vi "attenuation meter.vi"() -> ()   [LabVIEW 2014]
uses:
  Controls/App Data.ctl
  Controls/Main Enum.ctl
  <vilib>/Utility/NIReport.llb/NI_ReportGenerationCore.lvlib
  <resource>/objmgr/daqmx.rc
panel:
  in  "Erase all plots":bool
  out "Test results (spec.)":string
  in  "show test details":bool
  out "detailed results":string
  in  "Select TWT specification":string(combo)
  in  "auto measurement":bool
  in  "Number of cursors per plot":i32=4 min=2 max=4
  in  "plot 2 cursors visible?":bool=TRUE
  in  "plot 3 cursors visible?":bool=TRUE
  in  "plot 1 cursors visible?":bool=TRUE
  in  "Select plot":T1(radio)
  in  "Plot 3 color":u32(colorbox)=393471 caption="Plot 3"
  in  "Plot 2 color":u32(colorbox)=16716306 caption="Plot 2"
  in  "Plot 1 color":u32(colorbox) caption="Plot 1"
  in  "RF meter max.":dbl=10.1 min=0.0 max=500.0 format="%.2g"
  in  "RF meter min.":dbl=7.5 min=0.0 max=500.0 format="%.2g"
  in  "Batch":string="Batch: "
  in  "Run No":string="Run No: "
  in  "Date":string
  in  "Tube Type":string="Tube Type: "
  in  "Auto Record":bool
  in  "Device status":bool
  out "0 dB att. voltage (during last calibration)":dbl format="%.3g"
  out "Input voltages (updates \nonly when recording)":T2 {"Stop switch voltage" format="%.3g"; "Start switch voltage" format="%.3g"; "position voltage" format="%.3g"; "RF out voltage" format="%.3g"}
  in  "Re-calibrate 0dB":bool
  in  "Erase plot":bool
  in  "Record":bool
  in  "Print Button":bool
  in  "Select printer":string(combo)
  in  "minimum y [dB]":dbl=-1.0 min=-100.0 max=-0.1 step=0.1 format="%.1g"
  in  "averaging (1-10)":i32=5 min=1 max=10 step=1
  in  "ref. line [dB]":dbl=-0.09999999999999991 min=-5.0 max=0.0 step=0.01 format="%.3f"
  out "error out 2":errorcluster
  in  "error out":errorcluster
  out "XY Graph":T3(graph)
  # "Settings"
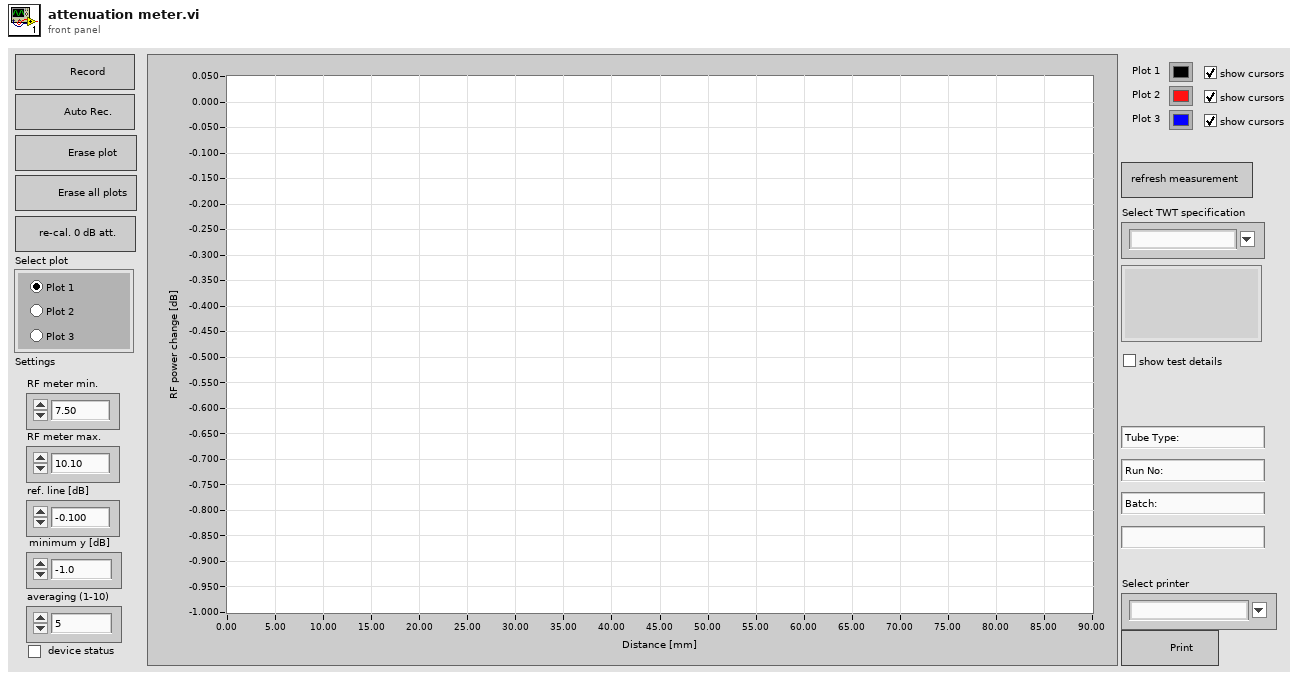
[diagram p1: front panel]
types:
  T1 = enum32{"Radio Selection 1", "Radio Selection 2", "Radio Selection 3"}
  T2 = cluster{"RF out voltage":dbl, "position voltage":dbl, "Start switch voltage":dbl, "Stop switch voltage":dbl}
  T3 = cluster{"plot 1 data":dbl[], "plot 1 data":dbl[]}[]
  T4 = typedef "Main Enum.ctl" = enum16{"Idle", "Initialize 1", "Initialize 2", "Initialize 3", "Calibrate RF output", "Update peaks colours", "Update anott. plots", "Save results", "Load results", "Erase plot", "Erase all plots", "Read new data", "Update plots", "Peak attenuation meas.", "Auto measurement", "Update cursors", "Update all cursors", "Print", "Check Start Stop triggers", "Plot 1 cursors visibility", "Plot 2 cursors visibility", "Plot 3 cursors visibility", "Error handler", "Exit", "Check results (spec.)"}
  T5 = typedef "App Data.ctl" = cluster{"DAQmx Task Name":refnum<k21>, "plot 0 data (ref.)":dbl[][], "plot 1 data":dbl[][], "plot 2 data":dbl[][], "plot 3 data":dbl[][], "Anott. plots":cluster{"plot 4 (anott.)":cluster{"x":dbl[], "y":dbl[]}, "plot 5 (anott.)":cluster{"x":dbl[], "y":dbl[]}, "plot 6 (anott.)":cluster{"x":dbl[], "y":dbl[]}}, "Active plot":u32, "Recording?":bool, "Cursors per plot":i32}
  T6 = enum16{"read", "write", "write number of cursors per plot only"}
  T7 = enum16{"get TWT types", "read TWT spec.", "save TWT spec."}
  T8 = enum8{"Enabled", "Disabled", "Disabled and Grayed Out"}
  T9 = enum16{"get TWT types", "read TWT spec.", "save TWT spec.", "remove TWT spec."}
  T10 = cluster{"plot 1 cursors visible? ":bool, "plot 2 cursors visible?":bool, "plot 3 cursors visible?":bool, "No of cursors per plot":i32}
  T11 = enum32{"invalid app kind", "Development System", "Run Time System", "Student Edition", "Embedded LabVIEW", "Evaluation", "Custom"}
  T12 = cluster{"plot 4 (anott.)":cluster{"x":dbl[], "y":dbl[]}, "plot 5 (anott.)":cluster{"x":dbl[], "y":dbl[]}, "plot 6 (anott.)":cluster{"x":dbl[], "y":dbl[]}}
  T13 = typedef "TWT spec..ctl" = cluster{"Reference level":dbl, "L1 min":dbl, "L1 max":dbl, "L2 min":dbl, "L2 max":dbl, "L3 min":dbl, "L3 max":dbl, "Tip loss nominal":dbl, "Tip loss min":dbl, "Tip loss max":dbl, "Centre loss nominal":dbl, "Centre loss min":dbl, "Centre loss max":dbl}
  T14 = cluster{"plot 3 data":dbl[], "plot 3 data":dbl[]}[]
  T15 = typedef "dist. between cursors.ctl" = cluster{"0 to c1":dbl, "c1 to c2":dbl, "c1 to c3":dbl, "c3 to c4":dbl}
  T16 = cluster{"Plot 1 distances":T15, "Plot 2 distances":T15, "Plot 3 distances":T15}
  T17 = cluster{"Tube Type":string, "Date":string, "Run No":string, "Batch":string}
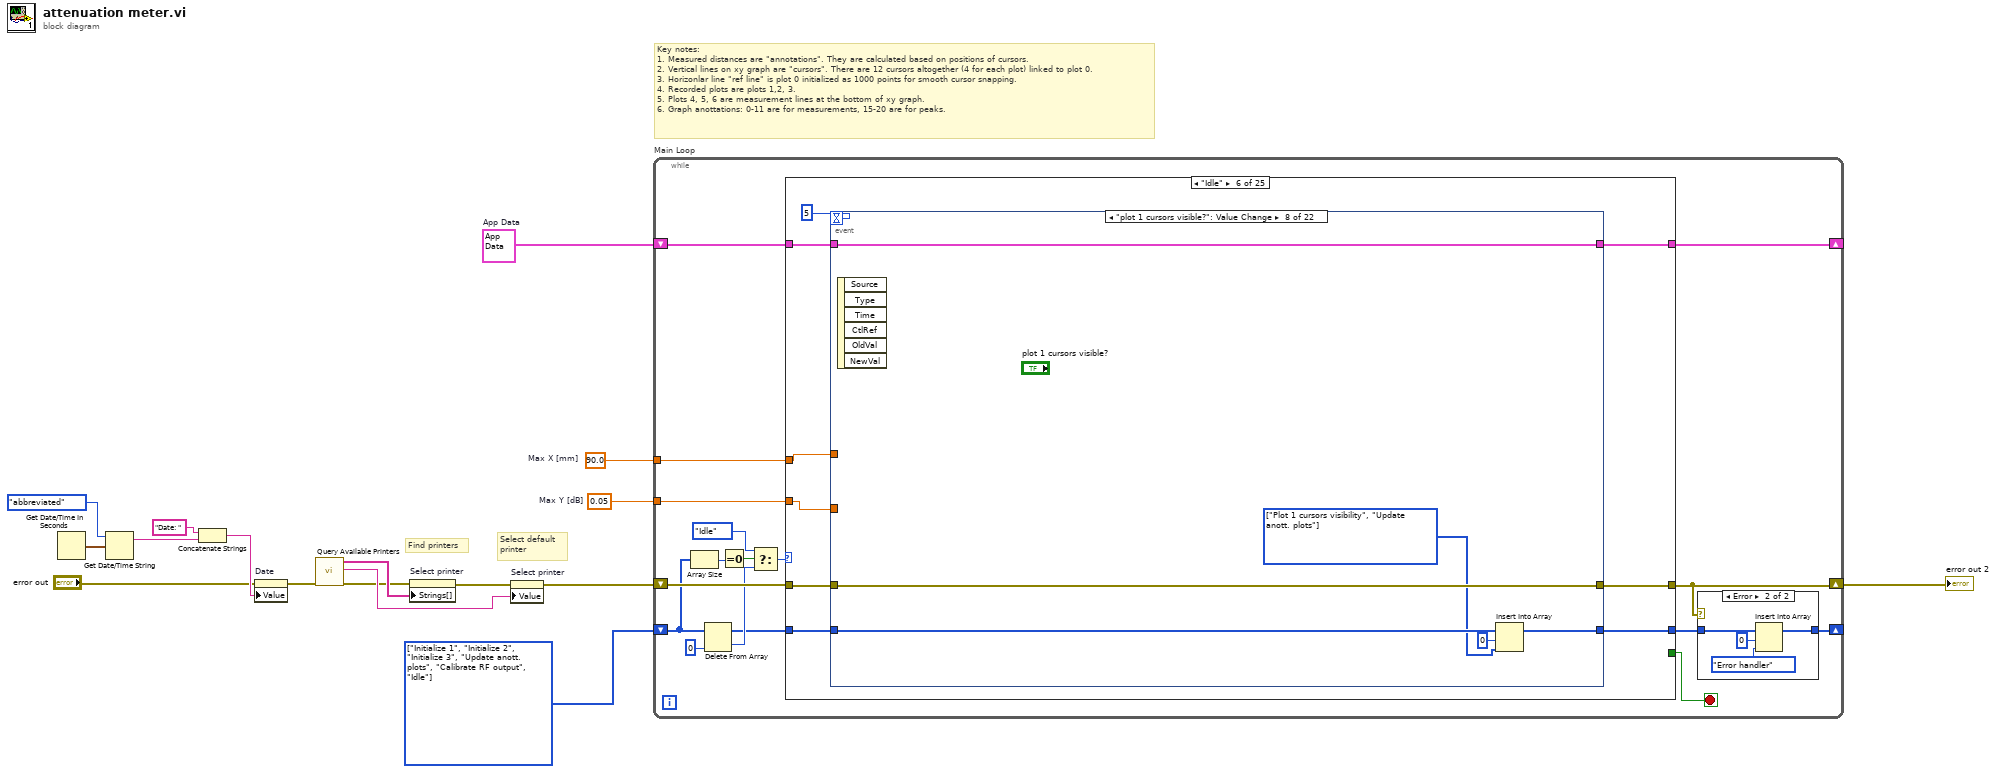
[diagram p0: block diagram]
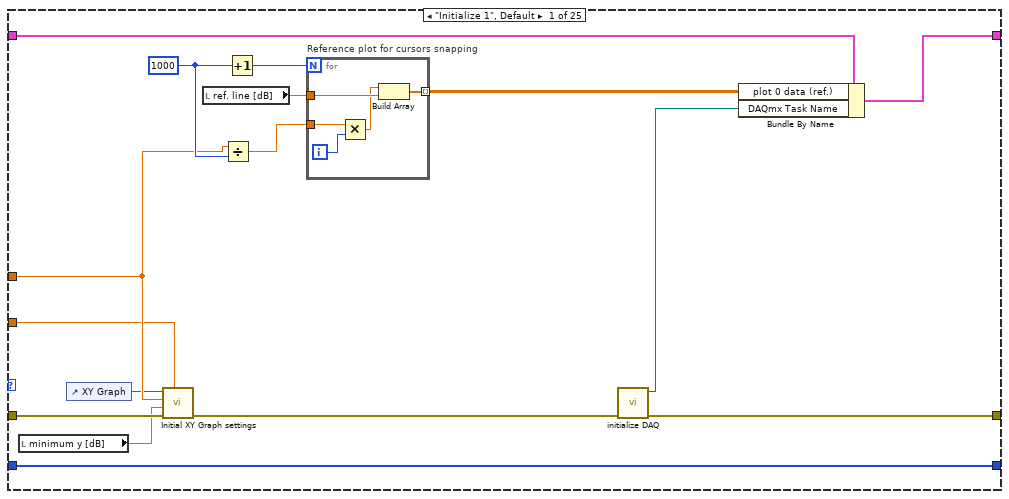
[diagram p3: hidden frame]
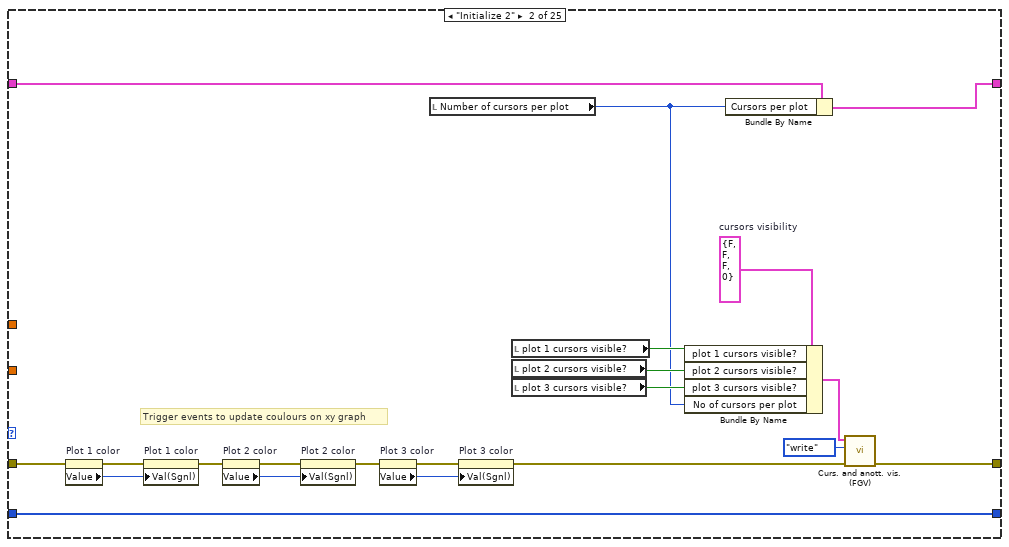
[diagram p4: hidden frame]
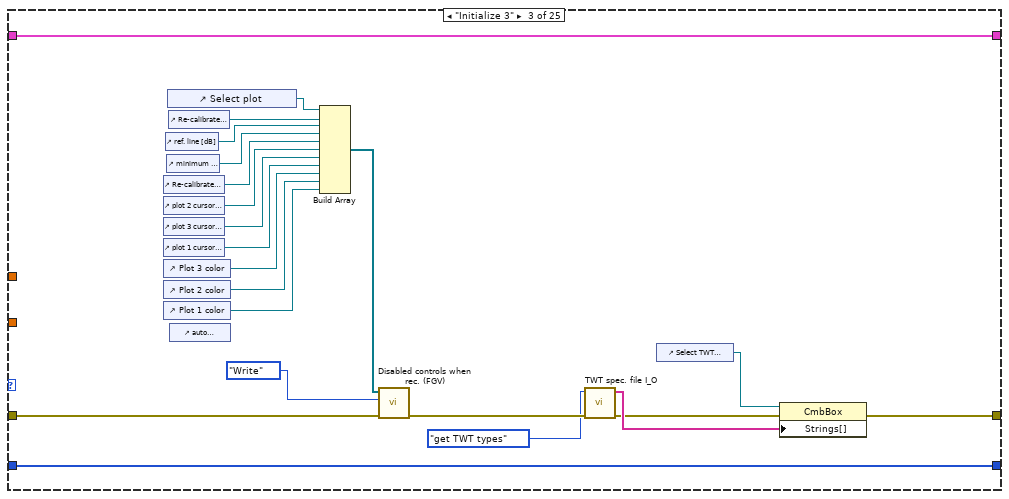
[diagram p5: hidden frame]
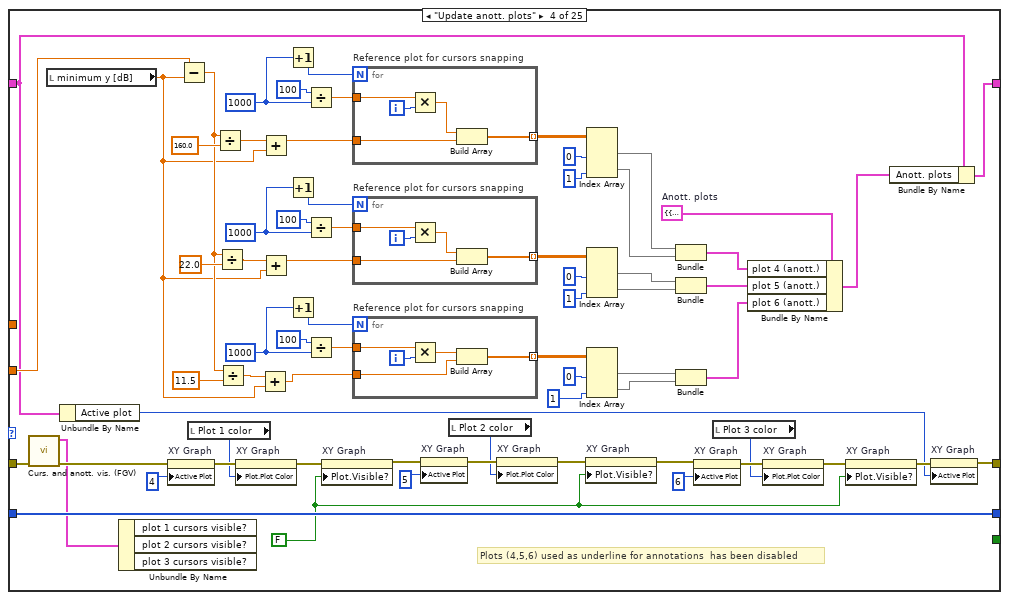
[diagram p6: hidden frame]
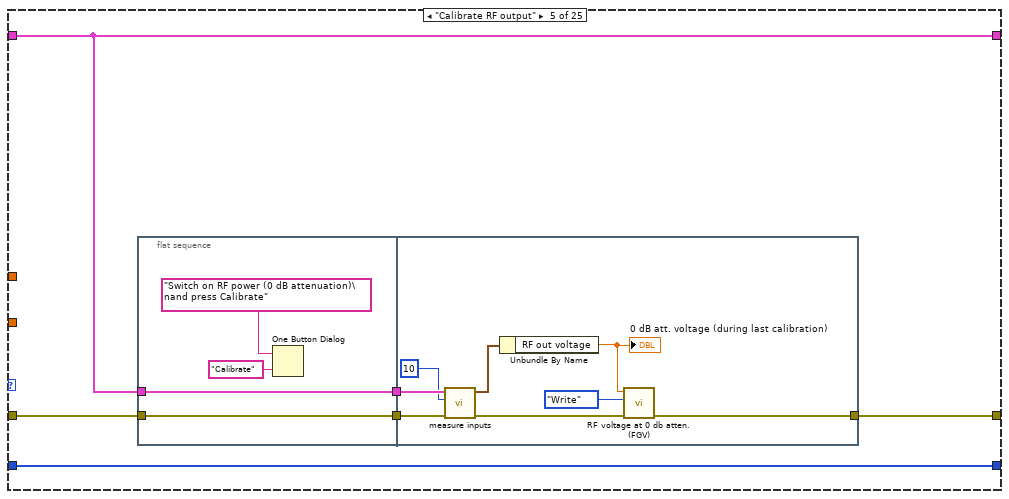
[diagram p7: hidden frame]
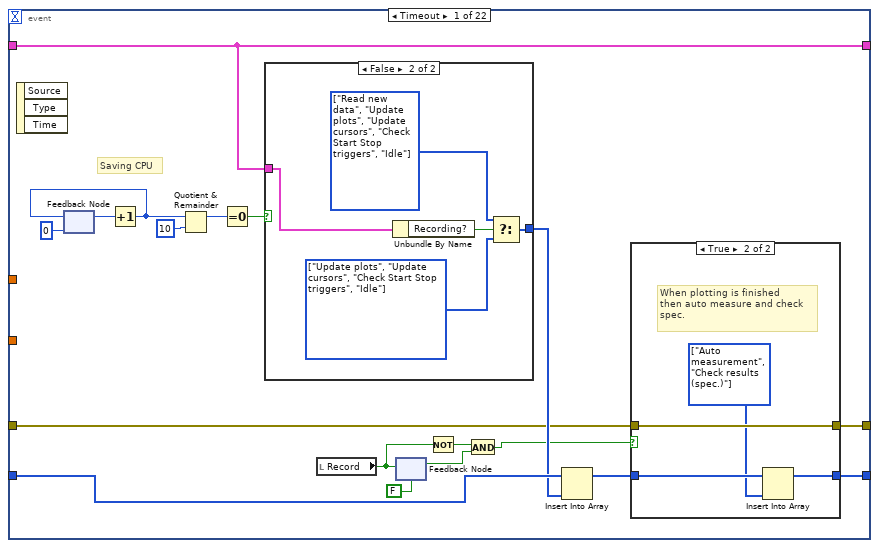
[diagram p8: hidden frame]
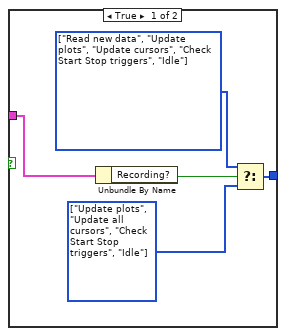
[diagram p10: hidden frame]
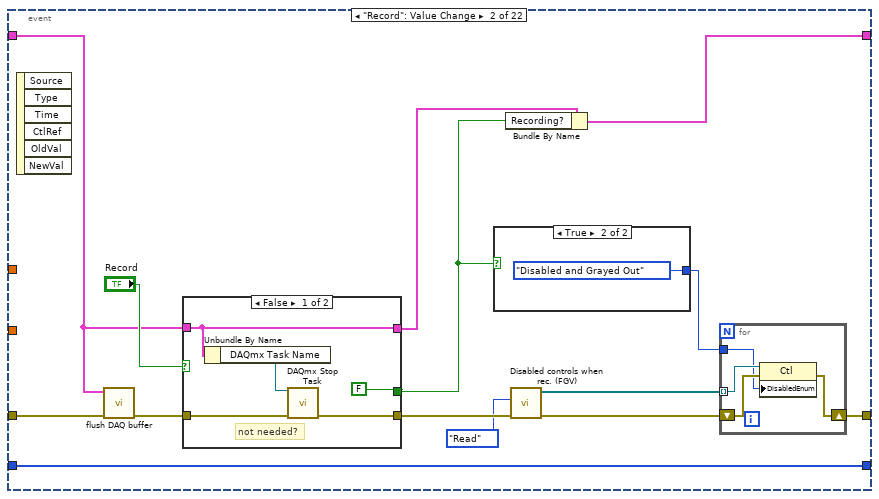
[diagram p11: hidden frame]
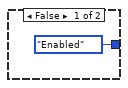
[diagram p12: hidden frame]
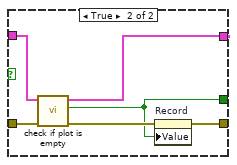
[diagram p13: hidden frame]
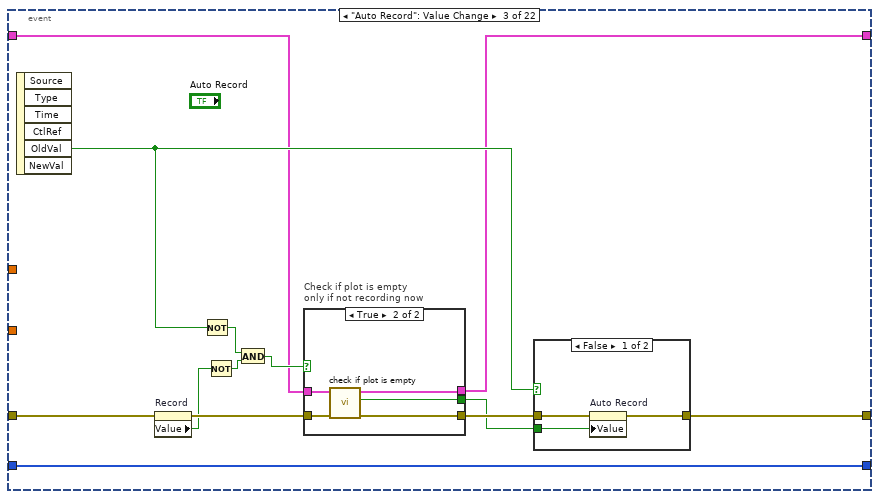
[diagram p14: hidden frame]
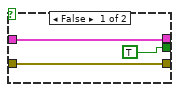
[diagram p15: hidden frame]
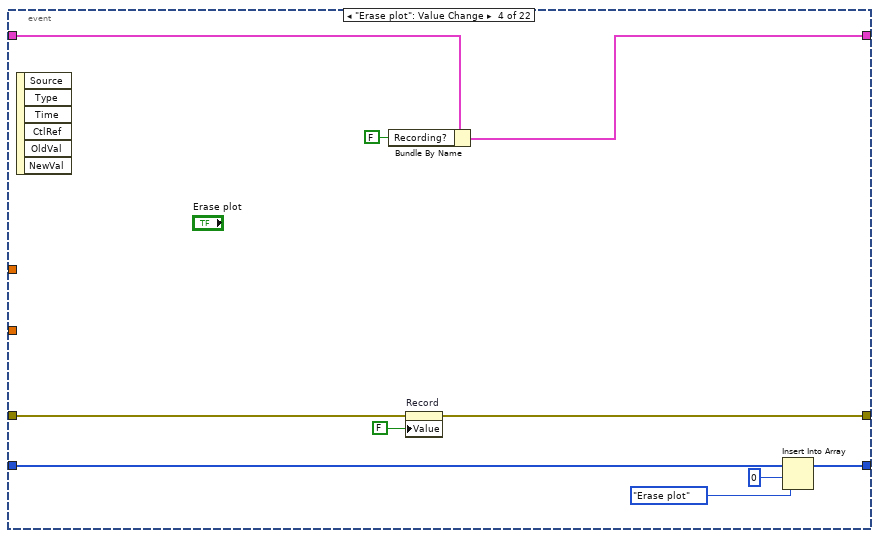
[diagram p17: hidden frame]
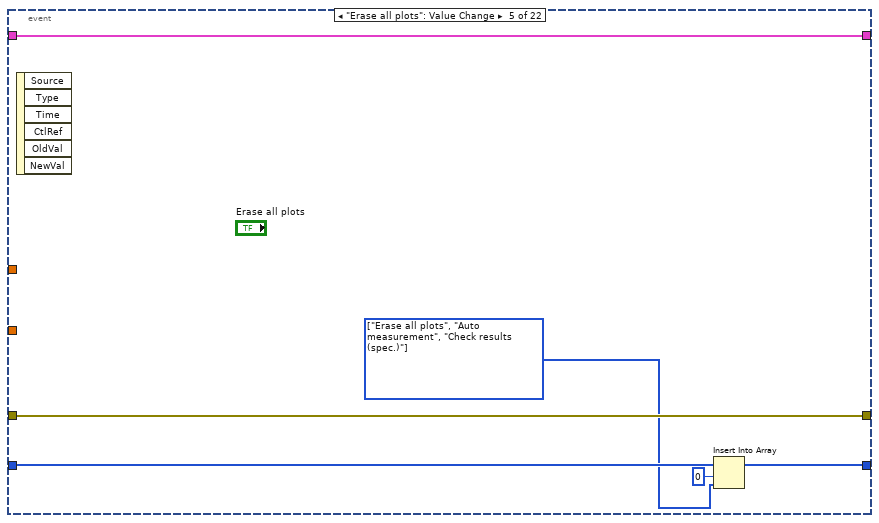
[diagram p18: hidden frame]
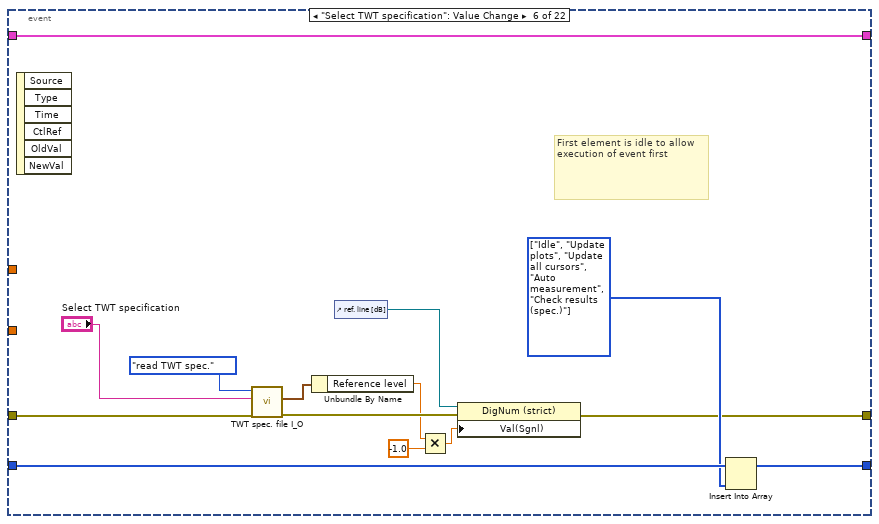
[diagram p19: hidden frame]
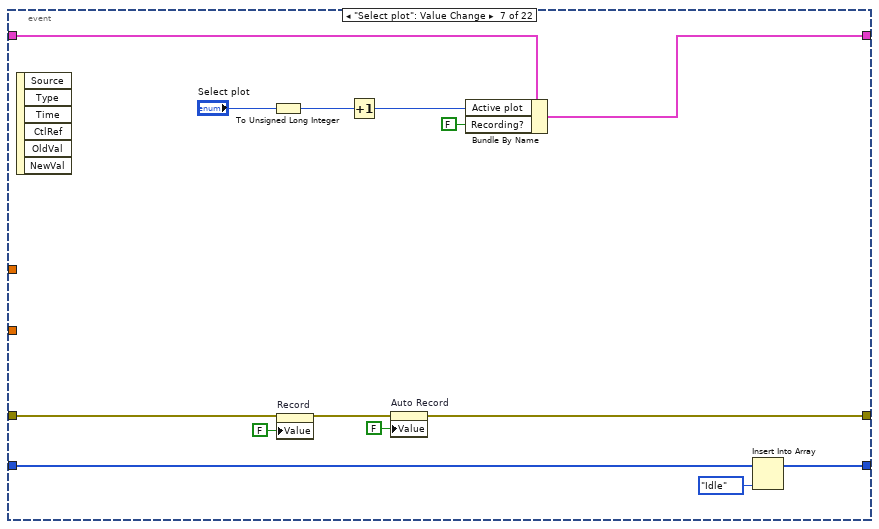
[diagram p20: hidden frame]
diagram:
  w2 = T4[] [enum."Initialize 1", enum."Initialize 2", enum."Initialize 3", enum."Update anott. plots", enum."Calibrate RF output", enum."Idle"] items=["Idle", "Initialize 1", "Initialize 2", "Initialize 3", "Calibrate RF output", "Update peaks colours", "Update anott. plots", "Save results", "Load results", "Erase plot", "Erase all plots", "Read new data", "Update plots", "Peak attenuation meas.", "Auto measurement", "Update cursors", "Update all cursors", "Print", "Check Start Stop triggers", "Plot 1 cursors visibility", "Plot 2 cursors visibility", "Plot 3 cursors visibility", "Error handler", "Exit", "Check results (spec.)"]
  w3 = 0.05  # Max Y [dB]
  w4 = T5 {"DAQmx Task Name"="", "plot 0 data (ref.)"=[], "plot 1 data"=[], "plot 2 data"=[], "plot 3 data"=[], "Anott. plots"={"plot 4 (anott.)"={"x"=[], "y"=[]}, "plot 5 (anott.)"={"x"=[], "y"=[]}, "plot 6 (anott.)"={"x"=[], "y"=[]}}, "Active plot"=1, "Recording?"=FALSE, "Cursors per plot"=4}  # App Data
  w16 = 90.0  # Max X [mm]
  # "Key notes:\n1. Measured distances are \"annotations\". They are calculated based on positions of cursors.\n2. Vertical lines on xy graph are \"cursors\". There are 12 cursors altogether (4 for each plot) linked to plot 0.\n3. Horizonlar line \"ref line\" is plot 0 initialized as 1000 points for smooth cursor snapping.\n4. Recorded plots are plots 1,2, 3.\n5. Plots 4, 5, 6 are measurement lines at the bottom of xy graph.\n6. Graph anottations: 0-11 are for measurements, 15-20 are for peaks."
  # "Select default \nprinter"
  # "Find printers"
  n1 = Get Date/Time In Seconds() -> (seconds since 1Jan1904=w6:timestamp)
  n2 = Get Date/Time String(date format (0)=enum16{"short", "long", "abbreviated"}."abbreviated", seconds (now)=w6) -> (date string=w9:string)  [unwired: 1 in, 1 out]
  n3 = Concatenate Strings("Date: " ("string"), w9) -> (w8:string)
  n4 = property on="Date" class="Str"(error in="error out", "Value"=w8) -> (error out=w5:errorcluster)  [unwired: 1 in, 1 out]
  n5 = call <vilib>:"Query Available Printers.vi"("error in (no error)"=w5) -> ("error out"=w12:errorcluster, "default printer"=w13:string, "system configured printers"=w15:string[])  [unwired: 8 in]
  n6 = property on="Select printer" class="CmbBox"(error in=w12, "Strings[]"=w15) -> (error out=w14:errorcluster)  [unwired: 1 in, 1 out]
  n7 = property on="Select printer" class="CmbBox"(error in=w14, "Value"=w13) -> (error out=w11:errorcluster)  [unwired: 1 in, 1 out]
  n8 = while "Main Loop" {
    shift-right: [w31] -> _
    shift-left: w4 -> [w34]
    shift-right: [w25] -> w17
    shift-left: w11 -> [w33]
    shift-right: [w26] -> _
    shift-left: w2 -> [w24]
    tunnel: w16 -> [w32]
    tunnel: w3 -> [w29]
    stop <- w30 stop-if-true
    n9 = Array Size(array=w24) -> (size(s)=w23:i32)
    n10 = Delete From Array(array=w24, index=0) -> (deleted portion=w21:T4, array with subset deleted=w18:T4[])  [unwired: 1 in]
    n11 = Equal To 0?(x=w23) -> (x = 0?=w22:bool)
    n12 = Select(t=Main_Enum."Idle", s=w22, f=w21) -> (s? t:f=w19:T4)
    n13 = case shown="\"Idle\"" w19 {
      tunnel: w34 -> [w55 w75 w101 w126 w192 w211 w504 w539 w552 w554 w566 w586 w631 w647 w653 w690 w693 w702 w711 w721 w724 w745 w765 w785 w793]
      tunnel: w33 -> [w53 w72 w89 w108 w189 w209 w507 w538 w551 w557 w582 w608 w632 w644 w650 w688 w695 w705 w713 w723 w727 w748 w767 w784 w794]
      tunnel: [w41 w76 w83 w110 w188 w210 w488 w537 w550 w556 w579 w594 w630 w637 w649 w681 w694 w704 w710 w717 w728 w746 w766 w784 w792] -> w25
      tunnel: [w54 w73 w101 w140 w192 w212 w505 w539 w552 w554 w566 w585 w631 w647 w654 w691 w693 w701 w711 w721 w724 w745 w765 w785 w793] -> w31
      tunnel: [_ _ _ _ _ _ _ _ _ _ _ _ _ _ _ _ _ _ _ TRUE _ _ _ _ _] -> w30
      tunnel: w32 -> [w48 _ _ _ _ w208 _ _ _ _ _ _ _ _ _ _ _ _ _ _ _ _ _ _ _]
      tunnel: w29 -> [w44 _ _ w139 _ w207 _ _ w547 w555 _ _ _ _ _ _ _ _ _ _ w725 w744 w764 _ _]
      tunnel: w18 -> [w40 w62 w88 w127 w187 w206 w496 w536 w541 w564 w565 w583 w633 w635 w651 w689 w692 w696 w709 w714 w726 w747 w768 w786 w788]
      tunnel: [w40 w62 w88 w127 w187 w205 w495 w536 w541 w564 w565 w583 w633 w635 w651 w689 w692 w696 w708 w714 w726 w747 w768 w786 w788] -> w27
      frame "Initialize 1", Default {
        w50 = 1000
        n14 = local read "minimum y [dB]"() -> (w46:dbl)
        n15 = control-ref of="XY Graph"() -> (w45:refnum<vi>)
        n16 = call "Initial XY Graph settings.vi"("Y Scale.Range:Maximum"=w44, "error in (no error)"=w53, "Y Minimum"=w46, "X Maximum"=w48, "XYGraph in"=w45) -> ("error out"=w52:errorcluster)  [unwired: 6 in]
        n17 = local read "ref. line [dB]"() -> (w51:dbl)
        n18 = Divide(x=w48, y=w50) -> (x/y=w49:dbl)
        n19 = Increment(x=w50) -> (x+1=w47:i32)
        n20 = for "Reference plot for cursors snapping" {
          N: w47 -> [_]
          tunnel: w51 -> [w59]
          tunnel: [w60] -> w43 mode=indexing
          tunnel: w49 -> [w57]
          i -> [w58]
          n21 = Multiply(x=w57, y=w58) -> (x*y=w56:dbl)
          n22 = Build Array(w56, w59) -> (w60:dbl[])
        }
        n23 = call "initialize DAQ.vi"("error in (no error)"=w52) -> ("error out"=w41:errorcluster, "Refnum out"=w42:refnum<k21>)  [unwired: 9 in]
        n24 = Bundle By Name(cluster=w55, "plot 0 data (ref.)"=w43, "DAQmx Task Name"=w42) -> (w54:T5)
      }
      frame "Initialize 2" {
        w78 = T10 {"plot 1 cursors visible? "=FALSE, "plot 2 cursors visible?"=FALSE, "plot 3 cursors visible?"=FALSE, "No of cursors per plot"=0}  # cursors visibility
        # "Trigger events to update coulours on xy graph"
        n25 = property on="Plot 1 color" class="ColBox"(error in=w72) -> (error out=w71:errorcluster, "Value"=w65:u32)  [unwired: 1 in, 1 out]
        n26 = property on="Plot 1 color" class="ColBox"(error in=w71, "Val(Sgnl)"=w65) -> (error out=w70:errorcluster)  [unwired: 1 in, 1 out]
        n27 = property on="Plot 2 color" class="ColBox"(error in=w70) -> (error out=w69:errorcluster, "Value"=w64:u32)  [unwired: 1 in, 1 out]
        n28 = property on="Plot 2 color" class="ColBox"(error in=w69, "Val(Sgnl)"=w64) -> (error out=w68:errorcluster)  [unwired: 1 in, 1 out]
        n29 = property on="Plot 3 color" class="ColBox"(error in=w68) -> (error out=w67:errorcluster, "Value"=w63:u32)  [unwired: 1 in, 1 out]
        n30 = local read "Number of cursors per plot"() -> (w74:i32)
        n31 = property on="Plot 3 color" class="ColBox"(error in=w67, "Val(Sgnl)"=w63) -> (error out=w66:errorcluster)  [unwired: 1 in, 1 out]
        n32 = local read "plot 1 cursors visible?"() -> (w81:bool)
        n33 = local read "plot 2 cursors visible?"() -> (w80:bool)
        n34 = local read "plot 3 cursors visible?"() -> (w79:bool)
        n35 = Bundle By Name(cluster=w78, "plot 1 cursors visible?"=w81, "plot 2 cursors visible?"=w80, "plot 3 cursors visible?"=w79, "No of cursors per plot"=w74) -> (w77:T10)
        n36 = Bundle By Name(cluster=w75, "Cursors per plot"=w74) -> (w73:T5)
        n37 = call "Curs. and anott. vis. (FGV).vi"("error in (no error)"=w66, "Enum"=T6."write", "cursors visibility in"=w77) -> ("error out"=w76:errorcluster)  [unwired: 6 in, 2 out]
      }
      frame "Initialize 3" {
        n38 = control-ref of="Re-calibrate 0dB"() -> (w98:refnum<vi>)
        n39 = control-ref of="plot 2 cursors visible?"() -> (w97:refnum<vi>)
        n40 = control-ref of="plot 3 cursors visible?"() -> (w96:refnum<vi>)
        n41 = control-ref of="plot 1 cursors visible?"() -> (w95:refnum<vi>)
        n42 = control-ref of="Plot 3 color"() -> (w94:refnum<vi>)
        n43 = control-ref of="Plot 2 color"() -> (w93:refnum<vi>)
        n44 = control-ref of="Plot 1 color"() -> (w92:refnum<vi>)
        n45 = control-ref of="ref. line [dB]"() -> (w100:refnum<vi>)
        n46 = control-ref of="minimum y [dB]"() -> (w99:refnum<vi>)
        n47 = control-ref of="Select plot"() -> (w102:refnum<vi>)
        n48 = control-ref of="Re-calibrate 0dB"() -> (w103:refnum<vi>)
        n49 = control-ref of="auto measurement"() -> ()  [unwired: 1 out]
        n50 = Build Array(w102, w103, w100, w99, w98, w97, w96, w95, w94, w93, w92) -> (w91:refnum<vi>[])
        n51 = call "Disabled controls when rec. (FGV) .vi"("error in (no error)"=w89, "Enum"=enum16{"Read", "Write"}."Write", "Array of controls"=w91) -> ("error out"=w87:errorcluster)  [unwired: 7 in, 1 out]
        n52 = call "TWT spec. file I_O.vi"("error in"=w87, "Enum"=T7."get TWT types") -> ("error out"=w82:errorcluster, "TWT types"=w84:string[])  [unwired: 7 in, 1 out]
        n53 = control-ref of="Select TWT specification"() -> (w85:refnum<vi>)
        n54 = property class="CmbBox"(reference=w85, error in=w82, "Strings[]"=w84) -> (error out=w83:errorcluster)  [unwired: 1 out]
      }
      frame "Update anott. plots" {
        w104 = FALSE ("Plot.Visible")
        w168 = T12 {"plot 4 (anott.)"={"x"=[], "y"=[]}, "plot 5 (anott.)"={"x"=[], "y"=[]}, "plot 6 (anott.)"={"x"=[], "y"=[]}}  # Anott. plots
        w164 = 1000
        w159 = 1000
        w155 = 1000
        # "Plots (4,5,6) used as underline for annotations  has been disabled"
        n55 = call "Curs. and anott. vis. (FGV).vi"("error in (no error)"=w108) -> ("error out"=w107:errorcluster, "cursors visibility out"=w106:T10)  [unwired: 8 in, 1 out]
        n56 = local read "minimum y [dB]"() -> (w128:dbl)
        n57 = Unbundle By Name(w126) -> ("Active plot"=w109:u32)
        n58 = Unbundle By Name(w106) -> ()  [unwired: 3 out]
        n59 = property on="XY Graph" class="XYGraph (strict)"(error in=w107, "Active Plot"=u32 4) -> (error out=w125:errorcluster)  [unwired: 1 in, 1 out]
        n60 = Subtract(x=w139, y=w128) -> (x-y=w133:dbl)
        n61 = local read "Plot 1 color"() -> (w122:u32)
        n62 = Divide(x=w133, y=160.0) -> (x/y=w137:dbl)
        n63 = Divide(x=w133, y=22.0 ("y 2")) -> (x/y=w135:dbl)
        n64 = Divide(x=w133, y=11.5 ("y 3")) -> (x/y=w129:dbl)
        n65 = property on="XY Graph" class="XYGraph (strict)"(error in=w125, "Plot.Plot Color"=w122) -> (error out=w123:errorcluster)  [unwired: 1 in, 1 out]
        n66 = Add(x=w129, y=w128) -> (x+y=w130:dbl)
        n67 = Add(x=w137, y=w128) -> (x+y=w132:dbl)
        n68 = Add(x=w135, y=w128) -> (x+y=w131:dbl)
        n69 = Increment(x=w155) -> (x+1=w153:i32)
        n70 = Increment(x=w159) -> (x+1=w161:i32)
        n71 = Increment(x=w164) -> (x+1=w162:i32)
        n72 = Divide(x=100, y=w155) -> (x/y=w154:dbl)
        n73 = Divide(x=100, y=w159) -> (x/y=w160:dbl)
        n74 = Divide(x=100, y=w164) -> (x/y=w163:dbl)
        n75 = property on="XY Graph" class="XYGraph (strict)"(error in=w123, "Plot.Visible?"=w104) -> (error out=w113:errorcluster)  [unwired: 1 in, 1 out]
        n76 = for "Reference plot for cursors snapping" {
          N: w153 -> [_]
          tunnel: w132 -> [w185]
          tunnel: [w186] -> w157 mode=indexing
          tunnel: w154 -> [w183]
          i -> [w184]
          n77 = Multiply(x=w183, y=w184) -> (x*y=w182:dbl)
          n78 = Build Array(w182, w185) -> (w186:dbl[])
        }
        n79 = for "Reference plot for cursors snapping" {
          N: w161 -> [_]
          tunnel: w131 -> [w180]
          tunnel: [w181] -> w167 mode=indexing
          tunnel: w160 -> [w178]
          i -> [w179]
          n80 = Multiply(x=w178, y=w179) -> (x*y=w177:dbl)
          n81 = Build Array(w177, w180) -> (w181:dbl[])
        }
        n82 = for "Reference plot for cursors snapping" {
          N: w162 -> [_]
          tunnel: w130 -> [w175]
          tunnel: [w176] -> w166 mode=indexing
          tunnel: w163 -> [w173]
          i -> [w174]
          n83 = Multiply(x=w173, y=w174) -> (x*y=w172:dbl)
          n84 = Build Array(w172, w175) -> (w176:dbl[])
        }
        n85 = property on="XY Graph" class="XYGraph (strict)"(error in=w113, "Active Plot"=u32 5) -> (error out=w119:errorcluster)  [unwired: 1 in, 1 out]
        n86 = local read "Plot 2 color"() -> (w115:u32)
        n87 = property on="XY Graph" class="XYGraph (strict)"(error in=w119, "Plot.Plot Color"=w115) -> (error out=w121:errorcluster)  [unwired: 1 in, 1 out]
        n88 = property on="XY Graph" class="XYGraph (strict)"(error in=w121, "Plot.Visible?"=w104) -> (error out=w114:errorcluster)  [unwired: 1 in, 1 out]
        n89 = Index Array(array=w157, index (col) #1=0 ("disabled index (col)"), index (col) #2=1 ("index (col)")) -> (element #1=w150:dbl[], element #2=w149:dbl[])  [unwired: 2 in]
        n90 = Index Array(array=w167, index (col) #1=0 ("disabled index (col)"), index (col) #2=1 ("index (col)")) -> (element #1=w147:dbl[], element #2=w148:dbl[])  [unwired: 2 in]
        n91 = Index Array(array=w166, index (col) #1=0 ("disabled index (col)"), index (col) #2=1 ("index (col)")) -> (element #1=w142:dbl[], element #2=w141:dbl[])  [unwired: 2 in]
        n92 = Bundle(w150, w149) -> (w169:cluster{dbl[], dbl[]})  [unwired: 1 in]
        n93 = Bundle(w147, w148) -> (w170:cluster{dbl[], dbl[]})  [unwired: 1 in]
        n94 = Bundle(w142, w141) -> (w171:cluster{dbl[], dbl[]})  [unwired: 1 in]
        n95 = property on="XY Graph" class="XYGraph (strict)"(error in=w114, "Active Plot"=u32 6) -> (error out=w118:errorcluster)  [unwired: 1 in, 1 out]
        n96 = local read "Plot 3 color"() -> (w112:u32)
        n97 = Bundle By Name(cluster=w168, "plot 4 (anott.)"=w169, "plot 5 (anott.)"=w170, "plot 6 (anott.)"=w171) -> (w105:T12)
        n98 = property on="XY Graph" class="XYGraph (strict)"(error in=w118, "Plot.Plot Color"=w112) -> (error out=w116:errorcluster)  [unwired: 1 in, 1 out]
        n99 = property on="XY Graph" class="XYGraph (strict)"(error in=w116, "Plot.Visible?"=w104) -> (error out=w111:errorcluster)  [unwired: 1 in, 1 out]
        n100 = Bundle By Name(cluster=w126, "Anott. plots"=w105) -> (w140:T5)
        n101 = property on="XY Graph" class="XYGraph (strict)"(error in=w111, "Active Plot"=w109) -> (error out=w110:errorcluster)  [unwired: 1 in, 1 out]
      }
      frame "Calibrate RF output" {
        n102 = flat-sequence {
          tunnel: w192 -> [w196]
          tunnel: [w196] -> w191
          tunnel: w189 -> [w193]
          tunnel: [w193] -> w190
          tunnel: w191 -> [w203]
          tunnel: w190 -> [w204]
          tunnel: [w199] -> w188
          frame #0 {
            n103 = One Button Dialog(message="Switch on RF power (0 dB attenuation)\nand press Calibrate", button name ("OK")="Calibrate") -> ()  [unwired: 1 out]
          }
          frame #1 {
            n104 = call "measure inputs.vi"("error in (no error)"=w204, "Sample averaging (1-10)"=10, "App Data"=w203) -> ("error out"=w200:errorcluster, "Analog inputs"=w201:T2)  [unwired: 7 in]
            n105 = Unbundle By Name(w201) -> ("RF out voltage"=w197:dbl)
            "0 dB att. voltage (during last calibration)" <- w197
            n106 = call "RF voltage at 0 db atten. (FGV).vi"("error in (no error)"=w200, "Enum"=enum16{"Read", "Write"}."Write", "RF voltage at 0 dB atten."=w197) -> ("error out"=w199:errorcluster)  [unwired: 7 in, 1 out]
          }
        }
      }
      frame "Idle" {
        n107 = event shown="[7] \"plot 1 cursors visible?\": Value Change" {
          selector: _ -> [_ _ _ _ _ _ _ _ _ _ _ _ _ _ _ _ _ _ _ _ _ _]
          dyn-events: _ -> [_ _ _ _ _ _ _ _ _ _ _ _ _ _ _ _ _ _ _ _ _ _]
          timeout: 5 -> [_ _ _ _ _ _ _ _ _ _ _ _ _ _ _ _ _ _ _ _ _ _]
          tunnel: [w231 w261 w280 w308 w319 w333 w346 w353 w359 w365 w376 w386 w395 w408 w421 w433 w441 w453 w468 w472 w480 w486] -> w212
          tunnel: w211 -> [w231 w248 w281 w309 w319 w333 w347 w353 w359 w365 w377 w386 w395 w408 w421 w433 w441 w454 w468 w472 w480 w486]
          tunnel: [w218 w255 w290 w312 w317 w323 w340 w352 w355 w361 w366 w383 w399 w402 w415 w427 w442 w455 w466 w473 w479 w485] -> w210
          tunnel: w209 -> [w219 w250 w288 w313 w317 w328 w342 w352 w355 w361 w368 w384 w398 w412 w424 w436 w442 w455 w467 w470 w479 w485]
          tunnel: w208 -> [_ _ _ _ _ _ _ _ _ _ _ _ _ _ _ _ _ w448 _ _ _ _]
          tunnel: w207 -> [_ _ _ _ _ _ _ _ _ _ _ _ _ _ _ _ _ _ _ _ _ _]
          tunnel: w206 -> [w230 w259 w279 w307 w318 w332 w336 w351 w357 w364 w375 w388 w400 w403 w413 w425 w440 w446 w461 w469 w477 w484]
          tunnel: [w220 w259 w279 w306 w316 w331 w335 w350 w358 w363 w374 w387 w400 w404 w414 w426 w439 w445 w462 w469 w478 w483] -> w205
          event Timeout {
            # "Saving CPU"
            n108 = event-data() -> ()  [unwired: 1 in, 3 out]
            n109 = feedback #1(0) -> (w227:i32)
            n110 = Increment(x=w227) -> (x+1=w226:i32)
            n111 = feedback-in #1(w226) -> ()
            n112 = Quotient & Remainder(x=w226, y=10) -> (x-y*floor(x/y)=w224:i32)  [unwired: 1 out]
            n113 = Equal To 0?(x=w224) -> (x = 0?=w223:bool)
            n114 = case shown="False" w223 {
              tunnel: w231 -> [w242 w247]
              tunnel: [w239 w244] -> w229
              frame True {
                w238 = T4[] [enum."Read new data", enum."Update plots", enum."Update cursors", enum."Check Start Stop triggers", enum."Idle"] items=["Idle", "Initialize 1", "Initialize 2", "Initialize 3", "Calibrate RF output", "Update peaks colours", "Update anott. plots", "Save results", "Load results", "Erase plot", "Erase all plots", "Read new data", "Update plots", "Peak attenuation meas.", "Auto measurement", "Update cursors", "Update all cursors", "Print", "Check Start Stop triggers", "Plot 1 cursors visibility", "Plot 2 cursors visibility", "Plot 3 cursors visibility", "Error handler", "Exit", "Check results (spec.)"]
                w240 = T4[] [enum."Update plots", enum."Update all cursors", enum."Check Start Stop triggers", enum."Idle"] items=["Idle", "Initialize 1", "Initialize 2", "Initialize 3", "Calibrate RF output", "Update peaks colours", "Update anott. plots", "Save results", "Load results", "Erase plot", "Erase all plots", "Read new data", "Update plots", "Peak attenuation meas.", "Auto measurement", "Update cursors", "Update all cursors", "Print", "Check Start Stop triggers", "Plot 1 cursors visibility", "Plot 2 cursors visibility", "Plot 3 cursors visibility", "Error handler", "Exit", "Check results (spec.)"]
                n115 = Unbundle By Name(w242) -> ("Recording?"=w241:bool)
                n116 = Select(t=w238, s=w241, f=w240) -> (s? t:f=w239:T4[])
              }
              frame False {
                w243 = T4[] [enum."Read new data", enum."Update plots", enum."Update cursors", enum."Check Start Stop triggers", enum."Idle"] items=["Idle", "Initialize 1", "Initialize 2", "Initialize 3", "Calibrate RF output", "Update peaks colours", "Update anott. plots", "Save results", "Load results", "Erase plot", "Erase all plots", "Read new data", "Update plots", "Peak attenuation meas.", "Auto measurement", "Update cursors", "Update all cursors", "Print", "Check Start Stop triggers", "Plot 1 cursors visibility", "Plot 2 cursors visibility", "Plot 3 cursors visibility", "Error handler", "Exit", "Check results (spec.)"]
                w245 = T4[] [enum."Update plots", enum."Update cursors", enum."Check Start Stop triggers", enum."Idle"] items=["Idle", "Initialize 1", "Initialize 2", "Initialize 3", "Calibrate RF output", "Update peaks colours", "Update anott. plots", "Save results", "Load results", "Erase plot", "Erase all plots", "Read new data", "Update plots", "Peak attenuation meas.", "Auto measurement", "Update cursors", "Update all cursors", "Print", "Check Start Stop triggers", "Plot 1 cursors visibility", "Plot 2 cursors visibility", "Plot 3 cursors visibility", "Error handler", "Exit", "Check results (spec.)"]
                n117 = Unbundle By Name(w247) -> ("Recording?"=w246:bool)
                n118 = Select(t=w243, s=w246, f=w245) -> (s? t:f=w244:T4[])
              }
            }
            n119 = local read "Record"() -> (w215:bool)
            n120 = feedback-in #2(w215) -> ()
            n121 = feedback #2(FALSE) -> (w214:bool)
            n122 = Not(x=w215) -> (.not. x?=w216:bool)
            n123 = And(x=w216, y=w214) -> (x .and. y?=w217:bool)
            n124 = Insert Into Array(array=w230, new element=w229) -> (w221:T4[])  [unwired: 1 in]
            n125 = case shown="True" w217 {
              tunnel: w221 -> [w232 w237]
              tunnel: [w232 w236] -> w220
              tunnel: w219 -> [w233 w235]
              tunnel: [w233 w235] -> w218
              frame False {
              }
              frame True {
                w234 = T4[] [enum."Auto measurement", enum."Check results (spec.)"] items=["Idle", "Initialize 1", "Initialize 2", "Initialize 3", "Calibrate RF output", "Update peaks colours", "Update anott. plots", "Save results", "Load results", "Erase plot", "Erase all plots", "Read new data", "Update plots", "Peak attenuation meas.", "Auto measurement", "Update cursors", "Update all cursors", "Print", "Check Start Stop triggers", "Plot 1 cursors visibility", "Plot 2 cursors visibility", "Plot 3 cursors visibility", "Error handler", "Exit", "Check results (spec.)"]
                # "When plotting is finished\nthen auto measure and check\nspec."
                n126 = Insert Into Array(array=w237, new element=w234) -> (w236:T4[])  [unwired: 1 in]
              }
            }
          }
          event "Record": Value Change {
            n127 = event-data() -> ()  [unwired: 1 in, 6 out]
            n128 = call "flush DAQ buffer.vi"("error in"=w250, "App Data"=w248) -> ("error out"=w249:errorcluster)  [unwired: 9 in]
            n129 = case shown="False" "Record" {
              tunnel: w249 -> [w270 w278]
              tunnel: w248 -> [w269 w277]
              tunnel: [w271 w275] -> w256
              tunnel: [FALSE ("record/overwrite?") w274] -> w252
              tunnel: [w269 w273] -> w260
              frame False {
                # "not needed?"
                n130 = Unbundle By Name(w269) -> ("DAQmx Task Name"=w268:refnum<k21>)
                n131 = call <vilib>:"DAQmx Stop Task.vi"("task/channels in"=w268, "error in"=w270) -> ("error out"=w271:errorcluster)  [unwired: 12 in, 1 out]
              }
              frame True {
                n132 = call "check if plot is empty.vi"("error in"=w278, "App Data in"=w277) -> ("error out"=w276:errorcluster, "record/overwrite?"=w274:bool, "App Data out"=w273:T5)  [unwired: 7 in]
                n133 = property on="Record" class="Bool (strict)"(error in=w276, "Value"=w274) -> (error out=w275:errorcluster)  [unwired: 1 in, 1 out]
              }
            }
            n134 = case shown="True" w252 {
              tunnel: [T8."Enabled" ("Disabled") T8."Disabled and Grayed Out" ("Disabled")] -> w253
              frame False {
              }
              frame True {
              }
            }
            n135 = Bundle By Name(cluster=w260, "Recording?"=w252) -> (w261:T5)
            n136 = call "Disabled controls when rec. (FGV) .vi"("error in (no error)"=w256, "Enum"=enum16{"Read", "Write"}."Read") -> ("error out"=w254:errorcluster, "Array of controls"=w257:refnum<vi>[])  [unwired: 8 in]
            n137 = for {
              tunnel: w257 -> [w267] mode=indexing
              shift-right: [w266] -> w255
              shift-left: w254 -> [w265]
              tunnel: w253 -> [w264]
              n138 = property class="Ctl"(reference=w267, error in=w265, "DisabledEnum"=w264) -> (error out=w266:errorcluster)  [unwired: 1 out]
            }
          }
          event "Auto Record": Value Change {
            n139 = event-data() -> ("OldVal"=w282:bool)  [unwired: 1 in, 5 out]
            n140 = property on="Record" class="Bool (strict)"(error in=w288) -> (error out=w287:errorcluster, "Value"=w286:bool)  [unwired: 1 in, 1 out]
            n141 = Not(x=w282) -> (.not. x?=w283:bool)
            n142 = Not(x=w286) -> (.not. x?=w285:bool)
            n143 = And(x=w283, y=w285) -> (x .and. y?=w284:bool)
            n144 = case "Check if plot is empty\nonly if not recording now" shown="True" w284 {
              tunnel: w287 -> [w293 w299]
              tunnel: w281 -> [w292 w298]
              tunnel: [w293 w297] -> w291
              tunnel: [TRUE ("record/overwrite?") w296] -> w289
              tunnel: [w292 w295] -> w280
              frame False {
              }
              frame True {
                n145 = call "check if plot is empty.vi"("error in"=w299, "App Data in"=w298) -> ("error out"=w297:errorcluster, "record/overwrite?"=w296:bool, "App Data out"=w295:T5)  [unwired: 7 in]
              }
            }
            n146 = case shown="False" w282 {
              tunnel: w291 -> [w302 w303]
              tunnel: [w301 w303] -> w290
              tunnel: w289 -> [w300 _]
              frame False {
                n147 = property on="Auto Record" class="Bool (strict)"(error in=w302, "Value"=w300) -> (error out=w301:errorcluster)  [unwired: 1 in, 1 out]
              }
              frame True {
              }
            }
          }
          event "Erase plot": Value Change {
            n148 = event-data() -> ()  [unwired: 1 in, 6 out]
            n149 = Bundle By Name(cluster=w309, "Recording?"=FALSE) -> (w308:T5)
            n150 = property on="Record" class="Bool (strict)"(error in=w313, "Value"=FALSE ("Value (Signaling)")) -> (error out=w312:errorcluster)  [unwired: 1 in, 1 out]
            n151 = Insert Into Array(array=w307, index=0, new element=Main_Enum."Erase plot" ("new element/subarray")) -> (w306:T4[])
          }
          event "Erase all plots": Value Change {
            w314 = T4[] [enum."Erase all plots", enum."Auto measurement", enum."Check results (spec.)"] items=["Idle", "Initialize 1", "Initialize 2", "Initialize 3", "Calibrate RF output", "Update peaks colours", "Update anott. plots", "Save results", "Load results", "Erase plot", "Erase all plots", "Read new data", "Update plots", "Peak attenuation meas.", "Auto measurement", "Update cursors", "Update all cursors", "Print", "Check Start Stop triggers", "Plot 1 cursors visibility", "Plot 2 cursors visibility", "Plot 3 cursors visibility", "Error handler", "Exit", "Check results (spec.)"]
            n152 = event-data() -> ()  [unwired: 1 in, 6 out]
            n153 = Insert Into Array(array=w318, index=0, new element=w314) -> (w316:T4[])
          }
          event "Select TWT specification": Value Change {
            w326 = T4[] [enum."Idle", enum."Update plots", enum."Update all cursors", enum."Auto measurement", enum."Check results (spec.)"] items=["Idle", "Initialize 1", "Initialize 2", "Initialize 3", "Calibrate RF output", "Update peaks colours", "Update anott. plots", "Save results", "Load results", "Erase plot", "Erase all plots", "Read new data", "Update plots", "Peak attenuation meas.", "Auto measurement", "Update cursors", "Update all cursors", "Print", "Check Start Stop triggers", "Plot 1 cursors visibility", "Plot 2 cursors visibility", "Plot 3 cursors visibility", "Error handler", "Exit", "Check results (spec.)"]
            # "First element is idle to allow execution of event first"
            n154 = event-data() -> ()  [unwired: 1 in, 6 out]
            n155 = call "TWT spec. file I_O.vi"("error in"=w328, "TWT type"="Select TWT specification", "Enum"=T9."read TWT spec.") -> ("error out"=w325:errorcluster, "TWT spec"=w327:T13)  [unwired: 6 in, 1 out]
            n156 = Unbundle By Name(w327) -> ("Reference level"=w322:dbl)
            n157 = control-ref of="ref. line [dB]"() -> (w324:refnum<vi>)
            n158 = Multiply(x=w322, y=-1.0) -> (x*y=w321:dbl)
            n159 = property class="DigNum (strict)"(reference=w324, error in=w325, "Val(Sgnl)"=w321) -> (error out=w323:errorcluster)  [unwired: 1 out]
            n160 = Insert Into Array(array=w332, new element=w326) -> (w331:T4[])  [unwired: 1 in]
          }
          event "Select plot": Value Change {
            n161 = event-data() -> ()  [unwired: 1 in, 6 out]
            n162 = To Unsigned Long Integer(number="Select plot") -> (unsigned 32bit integer=w344:u32)
            n163 = property on="Record" class="Bool (strict)"(error in=w342, "Value"=FALSE ("Record")) -> (error out=w341:errorcluster)  [unwired: 1 in, 1 out]
            n164 = Increment(x=w344) -> (x+1=w345:u32)
            n165 = property on="Auto Record" class="Bool (strict)"(error in=w341, "Value"=FALSE ("Auto Record")) -> (error out=w340:errorcluster)  [unwired: 1 in, 1 out]
            n166 = Bundle By Name(cluster=w347, "Active plot"=w345, "Recording?"=FALSE) -> (w346:T5)
            n167 = Insert Into Array(array=w336, new element=Main_Enum."Idle" ("new element/subarray")) -> (w335:T4[])  [unwired: 1 in]
          }
          event "plot 1 cursors visible?": Value Change {
            w348 = T4[] [enum."Plot 1 cursors visibility", enum."Update anott. plots"] items=["Idle", "Initialize 1", "Initialize 2", "Initialize 3", "Calibrate RF output", "Update peaks colours", "Update anott. plots", "Save results", "Load results", "Erase plot", "Erase all plots", "Read new data", "Update plots", "Peak attenuation meas.", "Auto measurement", "Update cursors", "Update all cursors", "Print", "Check Start Stop triggers", "Plot 1 cursors visibility", "Plot 2 cursors visibility", "Plot 3 cursors visibility", "Error handler", "Exit", "Check results (spec.)"]
            n168 = event-data() -> ()  [unwired: 1 in, 6 out]
            n169 = Insert Into Array(array=w351, index=0, new element=w348) -> (w350:T4[])
          }
          event "plot 2 cursors visible?": Value Change {
            w354 = T4[] [enum."Plot 2 cursors visibility", enum."Update anott. plots"] items=["Idle", "Initialize 1", "Initialize 2", "Initialize 3", "Calibrate RF output", "Update peaks colours", "Update anott. plots", "Save results", "Load results", "Erase plot", "Erase all plots", "Read new data", "Update plots", "Peak attenuation meas.", "Auto measurement", "Update cursors", "Update all cursors", "Print", "Check Start Stop triggers", "Plot 1 cursors visibility", "Plot 2 cursors visibility", "Plot 3 cursors visibility", "Error handler", "Exit", "Check results (spec.)"]
            n170 = event-data() -> ()  [unwired: 1 in, 6 out]
            n171 = Insert Into Array(array=w357, index=0, new element=w354) -> (w358:T4[])
          }
          event "plot 3 cursors visible?": Value Change {
            w360 = T4[] [enum."Plot 3 cursors visibility", enum."Update anott. plots"] items=["Idle", "Initialize 1", "Initialize 2", "Initialize 3", "Calibrate RF output", "Update peaks colours", "Update anott. plots", "Save results", "Load results", "Erase plot", "Erase all plots", "Read new data", "Update plots", "Peak attenuation meas.", "Auto measurement", "Update cursors", "Update all cursors", "Print", "Check Start Stop triggers", "Plot 1 cursors visibility", "Plot 2 cursors visibility", "Plot 3 cursors visibility", "Error handler", "Exit", "Check results (spec.)"]
            n172 = event-data() -> ()  [unwired: 1 in, 6 out]
            n173 = Insert Into Array(array=w364, index=0, new element=w360) -> (w363:T4[])
          }
          event "Number of cursors per plot": Value Change {
            w369 = T4[] [enum."Plot 1 cursors visibility", enum."Plot 2 cursors visibility", enum."Plot 3 cursors visibility"] items=["Idle", "Initialize 1", "Initialize 2", "Initialize 3", "Calibrate RF output", "Update peaks colours", "Update anott. plots", "Save results", "Load results", "Erase plot", "Erase all plots", "Read new data", "Update plots", "Peak attenuation meas.", "Auto measurement", "Update cursors", "Update all cursors", "Print", "Check Start Stop triggers", "Plot 1 cursors visibility", "Plot 2 cursors visibility", "Plot 3 cursors visibility", "Error handler", "Exit", "Check results (spec.)"]
            # "This event is no active (control is hidden)"
            n174 = event-data() -> ()  [unwired: 1 in, 6 out]
            n175 = Bundle By Name(cluster=T10 {"plot 1 cursors visible? "=FALSE, "plot 2 cursors visible?"=FALSE, "plot 3 cursors visible?"=FALSE, "No of cursors per plot"=0} ("cursors visibility in"), "No of cursors per plot"="Number of cursors per plot") -> (w370:T10)
            n176 = call "Curs. and anott. vis. (FGV).vi"("error in (no error)"=w368, "Enum"=T6."write number of cursors per plot only", "cursors visibility in"=w370) -> ("error out"=w367:errorcluster)  [unwired: 6 in, 2 out]
            n177 = Bundle By Name(cluster=w377, "Cursors per plot"="Number of cursors per plot") -> (w376:T5)
            n178 = disable-structure shown="Disabled" {
              disable-tunnel: w367 -> [w380 w381]
              disable-tunnel: [w379 w381] -> w366
              frame Disabled {
                n179 = control-ref of="XY Graph"() -> (w378:refnum<vi>)
                n180 = call "invisible cursors pos..vi"("error in (no error)"=w380, "XYGraph in"=w378) -> ("error out"=w379:errorcluster)  [unwired: 9 in]
              }
              frame Enabled {
              }
            }
            n181 = Insert Into Array(array=w375, new element=w369) -> (w374:T4[])  [unwired: 1 in]
          }
          event "auto measurement": Value Change {
            w382 = T4[] [enum."Auto measurement", enum."Update all cursors", enum."Check results (spec.)"] items=["Idle", "Initialize 1", "Initialize 2", "Initialize 3", "Calibrate RF output", "Update peaks colours", "Update anott. plots", "Save results", "Load results", "Erase plot", "Erase all plots", "Read new data", "Update plots", "Peak attenuation meas.", "Auto measurement", "Update cursors", "Update all cursors", "Print", "Check Start Stop triggers", "Plot 1 cursors visibility", "Plot 2 cursors visibility", "Plot 3 cursors visibility", "Error handler", "Exit", "Check results (spec.)"]
            n182 = event-data() -> ()  [unwired: 1 in, 6 out]
            n183 = case shown="True" "auto measurement" {
              tunnel: w388 -> [w390 w394]
              tunnel: [w390 w393] -> w387
              tunnel: w384 -> [w389 w392]
              tunnel: [w389 w392] -> w383
              tunnel: w382 -> [_ w391]
              frame False {
              }
              frame True {
                n184 = Insert Into Array(array=w394, new element=w391) -> (w393:T4[])  [unwired: 1 in]
              }
            }
          }
          event "show test details": Value Change {
            n185 = event-data() -> ()  [unwired: 1 in, 6 out]
            n186 = control-ref of="detailed results"() -> (w397:refnum<vi>)
            n187 = property class="Str"(reference=w397, error in=w398, "Visible"="show test details") -> (error out=w399:errorcluster)  [unwired: 1 out]
          }
          event "Plot 1 color": Value Change {
            w401 = T4[] [enum."Plot 1 cursors visibility", enum."Update anott. plots", enum."Update peaks colours"] items=["Idle", "Initialize 1", "Initialize 2", "Initialize 3", "Calibrate RF output", "Update peaks colours", "Update anott. plots", "Save results", "Load results", "Erase plot", "Erase all plots", "Read new data", "Update plots", "Peak attenuation meas.", "Auto measurement", "Update cursors", "Update all cursors", "Print", "Check Start Stop triggers", "Plot 1 cursors visibility", "Plot 2 cursors visibility", "Plot 3 cursors visibility", "Error handler", "Exit", "Check results (spec.)"]
            n188 = event-data() -> ()  [unwired: 1 in, 6 out]
            n189 = property on="XY Graph" class="XYGraph (strict)"(error in=w412, "Active Plot"=u32 1) -> (error out=w411:errorcluster)  [unwired: 1 in, 1 out]
            n190 = property on="XY Graph" class="XYGraph (strict)"(error in=w411, "Plot.Plot Color"="Plot 1 color") -> (error out=w406:errorcluster)  [unwired: 1 in, 1 out]
            n191 = Unbundle By Name(w408) -> ("Active plot"=w407:u32)
            n192 = property on="XY Graph" class="XYGraph (strict)"(error in=w406, "Active Plot"=w407) -> (error out=w402:errorcluster)  [unwired: 1 in, 1 out]
            n193 = Insert Into Array(array=w403, index=0, new element=w401) -> (w404:T4[])
          }
          event "Plot 2 color": Value Change {
            w416 = T4[] [enum."Plot 1 cursors visibility", enum."Update anott. plots", enum."Update peaks colours"] items=["Idle", "Initialize 1", "Initialize 2", "Initialize 3", "Calibrate RF output", "Update peaks colours", "Update anott. plots", "Save results", "Load results", "Erase plot", "Erase all plots", "Read new data", "Update plots", "Peak attenuation meas.", "Auto measurement", "Update cursors", "Update all cursors", "Print", "Check Start Stop triggers", "Plot 1 cursors visibility", "Plot 2 cursors visibility", "Plot 3 cursors visibility", "Error handler", "Exit", "Check results (spec.)"]
            n194 = event-data() -> ()  [unwired: 1 in, 6 out]
            n195 = property on="XY Graph" class="XYGraph (strict)"(error in=w424, "Active Plot"=u32 2) -> (error out=w423:errorcluster)  [unwired: 1 in, 1 out]
            n196 = property on="XY Graph" class="XYGraph (strict)"(error in=w423, "Plot.Plot Color"="Plot 2 color") -> (error out=w419:errorcluster)  [unwired: 1 in, 1 out]
            n197 = Unbundle By Name(w421) -> ("Active plot"=w420:u32)
            n198 = property on="XY Graph" class="XYGraph (strict)"(error in=w419, "Active Plot"=w420) -> (error out=w415:errorcluster)  [unwired: 1 in, 1 out]
            n199 = Insert Into Array(array=w413, index=0, new element=w416) -> (w414:T4[])
          }
          event "Plot 3 color": Value Change {
            w428 = T4[] [enum."Plot 1 cursors visibility", enum."Update anott. plots", enum."Update peaks colours"] items=["Idle", "Initialize 1", "Initialize 2", "Initialize 3", "Calibrate RF output", "Update peaks colours", "Update anott. plots", "Save results", "Load results", "Erase plot", "Erase all plots", "Read new data", "Update plots", "Peak attenuation meas.", "Auto measurement", "Update cursors", "Update all cursors", "Print", "Check Start Stop triggers", "Plot 1 cursors visibility", "Plot 2 cursors visibility", "Plot 3 cursors visibility", "Error handler", "Exit", "Check results (spec.)"]
            n200 = event-data() -> ()  [unwired: 1 in, 6 out]
            n201 = property on="XY Graph" class="XYGraph (strict)"(error in=w436, "Active Plot"=u32 3) -> (error out=w435:errorcluster)  [unwired: 1 in, 1 out]
            n202 = property on="XY Graph" class="XYGraph (strict)"(error in=w435, "Plot.Plot Color"="Plot 3 color") -> (error out=w431:errorcluster)  [unwired: 1 in, 1 out]
            n203 = Unbundle By Name(w433) -> ("Active plot"=w432:u32)
            n204 = property on="XY Graph" class="XYGraph (strict)"(error in=w431, "Active Plot"=w432) -> (error out=w427:errorcluster)  [unwired: 1 in, 1 out]
            n205 = Insert Into Array(array=w425, index=0, new element=w428) -> (w426:T4[])
          }
          event "Re-calibrate 0dB": Value Change {
            w437 = T4[] [enum."Erase plot", enum."Calibrate RF output"] items=["Idle", "Initialize 1", "Initialize 2", "Initialize 3", "Calibrate RF output", "Update peaks colours", "Update anott. plots", "Save results", "Load results", "Erase plot", "Erase all plots", "Read new data", "Update plots", "Peak attenuation meas.", "Auto measurement", "Update cursors", "Update all cursors", "Print", "Check Start Stop triggers", "Plot 1 cursors visibility", "Plot 2 cursors visibility", "Plot 3 cursors visibility", "Error handler", "Exit", "Check results (spec.)"]
            n206 = event-data() -> ()  [unwired: 1 in, 6 out]
            n207 = Insert Into Array(array=w440, index=0, new element=w437) -> (w439:T4[])
          }
          event "ref. line [dB]": Value Change {
            w443 = T4[] [enum."Update plots", enum."Update all cursors"] items=["Idle", "Initialize 1", "Initialize 2", "Initialize 3", "Calibrate RF output", "Update peaks colours", "Update anott. plots", "Save results", "Load results", "Erase plot", "Erase all plots", "Read new data", "Update plots", "Peak attenuation meas.", "Auto measurement", "Update cursors", "Update all cursors", "Print", "Check Start Stop triggers", "Plot 1 cursors visibility", "Plot 2 cursors visibility", "Plot 3 cursors visibility", "Error handler", "Exit", "Check results (spec.)"]
            w452 = 1000
            n208 = event-data() -> ()  [unwired: 1 in, 6 out]
            n209 = Divide(x=w448, y=w452) -> (x/y=w451:dbl)
            n210 = Increment(x=w452) -> (x+1=w450:i32)
            n211 = for "Reference line" {
              N: w450 -> [_]
              tunnel: "ref. line [dB]" -> [w459]
              tunnel: [w460] -> w447 mode=indexing
              tunnel: w451 -> [w457]
              i -> [w458]
              n212 = Multiply(x=w457, y=w458) -> (x*y=w456:dbl)
              n213 = Build Array(w456, w459) -> (w460:dbl[])
            }
            n214 = Bundle By Name(cluster=w454, "plot 0 data (ref.)"=w447) -> (w453:T5)
            n215 = Insert Into Array(array=w446, index=0, new element=w443) -> (w445:T4[])
          }
          event "minimum y [dB]": Value Change {
            w463 = T4[] [enum."Update plots", enum."Update anott. plots", enum."Update all cursors"] items=["Idle", "Initialize 1", "Initialize 2", "Initialize 3", "Calibrate RF output", "Update peaks colours", "Update anott. plots", "Save results", "Load results", "Erase plot", "Erase all plots", "Read new data", "Update plots", "Peak attenuation meas.", "Auto measurement", "Update cursors", "Update all cursors", "Print", "Check Start Stop triggers", "Plot 1 cursors visibility", "Plot 2 cursors visibility", "Plot 3 cursors visibility", "Error handler", "Exit", "Check results (spec.)"]
            n216 = event-data() -> ()  [unwired: 1 in, 6 out]
            n217 = property on="XY Graph" class="XYGraph (strict)"(error in=w467, "YScale.Minimum"="minimum y [dB]") -> (error out=w466:errorcluster)  [unwired: 1 in, 1 out]
            n218 = Insert Into Array(array=w461, index=0, new element=w463) -> (w462:T4[])
          }
          event "Device status": Value Change {
            n219 = event-data() -> ()  [unwired: 1 in, 6 out]
            n220 = property on="Input voltages (updates \nonly when recording)" class="Clust (strict)"(error in=w470, "Visible"="Device status") -> (error out=w474:errorcluster)  [unwired: 1 in, 1 out]
            n221 = property on="0 dB att. voltage (during last calibration)" class="DigNum (strict)"(error in=w474, "Visible"="Device status") -> (error out=w473:errorcluster)  [unwired: 1 in, 1 out]
          }
          event "Print Button": Value Change {
            n222 = event-data() -> ()  [unwired: 1 in, 6 out]
            n223 = Insert Into Array(array=w477, index=0, new element=Main_Enum."Print") -> (w478:T4[])
          }
          event Panel Close? {
            n224 = event-data() -> ()  [unwired: 1 in, 4 out]
            n225 = Insert Into Array(array=w484, index=0, new element=Main_Enum."Exit") -> (w483:T4[])
            n226 = event-data("Discard?"=TRUE) -> ()  [unwired: 1 in, 1 out]
          }
        }
      }
      frame "Read new data" {
        n227 = Unbundle By Name(w504) -> ("Active plot"=w506:u32, "DAQmx Task Name"=w493:refnum<k21>)
        n228 = call "measure inputs.vi"("error in (no error)"=w507, "Sample averaging (1-10)"="averaging (1-10)", "App Data"=w504) -> ("error out"=w499:errorcluster, "Analog inputs"=w500:T2)  [unwired: 7 in]
        "Input voltages (updates \nonly when recording)" <- w500
        n229 = call "Voltage_inputs to x_y_scales.vi"("error in (no error)"=w499, "RF meter max."="RF meter max.", "RF meter min."="RF meter min.", "Analog inputs"=w500) -> ("error out"=w494:errorcluster, "y axis value"=w501:dbl, "x axis value"=w502:dbl)  [unwired: 5 in]
        n230 = property class="DAQmx Read"(reference=w493, error in=w494) -> (error out=w489:errorcluster, "AvailSampPerChan"=w492:u32)  [unwired: 1 out]
        n231 = case shown="3" w506 {
          tunnel: w504 -> [w517 w524 w531]
          tunnel: w501 -> [w519 w526 w533]
          tunnel: w502 -> [w518 w525 w532]
          tunnel: [w515 w522 w529] -> w505
          frame 1, Default {
            n232 = Unbundle By Name(w517) -> ("plot 1 data"=w521:dbl[][])
            n233 = Build Array(w518, w519) -> (w520:dbl[])
            n234 = Build Array (concatenate)(w521, w520) -> (w516:dbl[][])
            n235 = Bundle By Name(cluster=w517, "plot 1 data"=w516) -> (w515:T5)
          }
          frame 2 {
            n236 = Unbundle By Name(w524) -> ("plot 2 data"=w528:dbl[][])
            n237 = Build Array(w525, w526) -> (w527:dbl[])
            n238 = Build Array (concatenate)(w528, w527) -> (w523:dbl[][])
            n239 = Bundle By Name(cluster=w524, "plot 2 data"=w523) -> (w522:T5)
          }
          frame 3 {
            n240 = Unbundle By Name(w531) -> ("plot 3 data"=w535:dbl[][])
            n241 = Build Array(w532, w533) -> (w534:dbl[])
            n242 = Build Array (concatenate)(w535, w534) -> (w530:dbl[][])
            n243 = Bundle By Name(cluster=w531, "plot 3 data"=w530) -> (w529:T5)
          }
        }
        n244 = Greater?(x=w492, y=u32 20) -> (0:w490:bool)
        n245 = case shown="True" w490 {
          tunnel: w496 -> [w508 w514]
          tunnel: [w508 w513] -> w495
          tunnel: w489 -> [w509 w510]
          tunnel: [w509 w510] -> w488
          frame False {
          }
          frame True {
            n246 = Insert Into Array "Insert Into Array"(array=w514, index=0, new element=Main_Enum."Read new data" ("new element/subarray")) -> (w513:T4[])
          }
        }
      }
      frame "Update plots" {
        n247 = call "XY data formatting.vi"("error in (no error)"=w538, "App Data"=w539) -> ("error out"=w537:errorcluster, "Array"=→"XY Graph":T14)  [unwired: 8 in]
      }
      frame "Update cursors" {
        n248 = local read "minimum y [dB]"() -> (w548:dbl)
        n249 = control-ref of="XY Graph"() -> (w549:refnum<vi>)
        n250 = call "Calculate cursors' distances.vi"("error in (no error)"=w551, "XY Graph"=w549) -> ("error out"=w546:errorcluster, "All cursors' dist."=w543:T16)  [unwired: 8 in]
        n251 = call "Select annot. for update.vi"("error in"=w546, "All cursors' dist."=w543) -> ("error out"=w545:errorcluster, "Anott. for update"=w542:i32[], "All cursors' dist."=w544:T16)  [unwired: 7 in]
        n252 = call "Update distance annotations.vi"("Y axis max"=w547, "Y axis min"=w548, "error in (no error)"=w545, "Anott. for update array in"=w542, "All cursors' dist."=w544, "XY Graph"=w549) -> ("error out"=w550:errorcluster)  [unwired: 5 in]
      }
      frame "Update all cursors" {
        w553 = i32[] [0, 1, 2, 3, 4, 5, 6, 7, 8, 9, 10, 11, 12]  # all anottations
        n253 = local read "minimum y [dB]"() -> (w562:dbl)
        n254 = control-ref of="XY Graph"() -> (w563:refnum<vi>)
        n255 = call "Calculate cursors' distances.vi"("error in (no error)"=w557, "XY Graph"=w563) -> ("error out"=w561:errorcluster, "All cursors' dist."=w558:T16)  [unwired: 8 in]
        n256 = call "Select annot. for update.vi"("error in"=w561, "All cursors' dist."=w558) -> ("error out"=w560:errorcluster, "All cursors' dist."=w559:T16)  [unwired: 7 in, 1 out]
        n257 = call "Update distance annotations.vi"("Y axis max"=w555, "Y axis min"=w562, "error in (no error)"=w560, "Anott. for update array in"=w553, "All cursors' dist."=w559, "XY Graph"=w563) -> ("error out"=w556:errorcluster)  [unwired: 5 in]
      }
      frame "Update peaks colours" {
        w567 = 2  # Number of peak anott.
        w568 = 19  # starting index
        w569 = 2  # Number of peak anott.
        w570 = 17  # starting index
        w571 = 2  # Number of peak anott.
        w572 = 15  # starting index
        # "Update all(?) peak colours. Add this case in colour change events"
        n258 = local read "Plot 1 color"() -> (w578:u32)
        n259 = control-ref of="XY Graph"() -> (w573:refnum<vi>)
        n260 = call "update peak anott. colour.vi"("Color"=w578, "error in"=w582, "Number of peak anott."=w571, "starting index"=w572, "XY Graph"=w573) -> ("error out"=w581:errorcluster, "XY Graph out"=w575:refnum<vi>)  [unwired: 5 in]
        n261 = local read "Plot 2 color"() -> (w577:u32)
        n262 = call "update peak anott. colour.vi"("Color"=w577, "error in"=w581, "Number of peak anott."=w569, "starting index"=w570, "XY Graph"=w575) -> ("error out"=w580:errorcluster, "XY Graph out"=w574:refnum<vi>)  [unwired: 5 in]
        n263 = local read "Plot 3 color"() -> (w576:u32)
        n264 = call "update peak anott. colour.vi"("Color"=w576, "error in"=w580, "Number of peak anott."=w567, "starting index"=w568, "XY Graph"=w574) -> ("error out"=w579:errorcluster)  [unwired: 5 in, 1 out]
      }
      frame "Check Start Stop triggers" {
        # "Delay is for switch \ndebouncing"
        n265 = call "measure inputs.vi"("error in (no error)"=w608, "Sample averaging (1-10)"=1, "App Data"=w586) -> ("error out"=w597:errorcluster, "Analog inputs"=w607:T2)  [unwired: 7 in]
        n266 = Unbundle By Name(w586) -> ("Recording?"=w592:bool)
        n267 = Unbundle By Name(w607) -> ("Stop switch voltage"=w595:dbl, "Start switch voltage"=w604:dbl)
        n268 = local read "Auto Record"() -> (w584:bool)
        n269 = feedback #3(0.0 ("Start switch voltage")) -> (w599:dbl)
        n270 = feedback-in #3(w595) -> ()
        n271 = feedback-in #4(w604) -> ()
        n272 = feedback #4(0.0 ("Start switch voltage")) -> (w605:dbl)
        n273 = Subtract(x=w595, y=w599) -> (x-y=w600:dbl)
        n274 = Subtract(x=w604, y=w605) -> (x-y=w603:dbl)
        n275 = Greater? "Stop edge?"(x=w600, y=2.1) -> (0:w591:bool)
        n276 = Greater? "Start edge?"(x=w603, y=2.5) -> (0:w589:bool)
        n277 = And(x=w584, y=w589) -> (x .and. y?=w588:bool)
        n278 = Compound Arithmetic op=AND(w592, w591, w584) -> (w590:bool)
        n279 = case shown="False" w588 {
          tunnel: w597 -> [w621 w626]
          tunnel: [w621 w627] -> w593
          tunnel: w586 -> [w620 w624]
          tunnel: [w620 w622] -> w587
          frame False {
          }
          frame True {
            n280 = Bundle By Name(cluster=w624, "Recording?"=TRUE) -> (w622:T5)
            n281 = property on="Record" class="Bool (strict)"(error in=w626, "Value"=TRUE ("Value (Signaling)")) -> (error out=w627:errorcluster)  [unwired: 1 in, 1 out]
          }
        }
        n282 = case shown="True" w590 {
          tunnel: w593 -> [w610 w615]
          tunnel: [w610 w611] -> w594
          tunnel: w587 -> [w609 w618]
          tunnel: [w609 w616] -> w585
          frame False {
          }
          frame True {
            n283 = Bundle By Name(cluster=w618, "Recording?"=FALSE) -> (w616:T5)
            n284 = property on="Auto Record" class="Bool (strict)"(error in=w615, "Value"=FALSE ("Auto Record")) -> (error out=w612:errorcluster)  [unwired: 1 in, 1 out]
            n285 = property on="Record" class="Bool (strict)"(error in=w615, "Value"=FALSE ("Value (Signaling)")) -> (error out=w613:errorcluster)  [unwired: 1 in, 1 out]
            n286 = Merge Errors(w612, w613) -> (w611:errorcluster)
          }
        }
      }
      frame "Auto measurement" {
        n287 = control-ref of="XY Graph"() -> (w628:refnum<vi>)
        n288 = local read "ref. line [dB]"() -> (w629:dbl)
        n289 = call "auto measurement.vi"("ref. line [dB]"=w629, "error in"=w632, "App Data"=w631, "XYGraph in"=w628) -> ("error out"=w630:errorcluster)  [unwired: 7 in]
      }
      frame "Print" {
        # "Remove \"cancel\" error"
        n290 = local read "XY Graph"() -> (w643:T3)
        n291 = local read "Test results (spec.)"() -> (w634:string)
        n292 = control-ref of="XY Graph"() -> (w636:refnum<vi>)
        n293 = Bundle("Tube Type"="Tube Type", "Date"="Date", "Run No"="Run No", "Batch"="Batch") -> (w638:T17)  [unwired: 1 in]
        n294 = call "printout panel.vi"("Test results (spec.)"=w634, "Print add. info"=w638, "error in (no error)"=w644, "print data"=w643, "selected printer"="Select printer", "XY Graph (main VI)"=w636) -> ("error out"=w646:errorcluster)  [unwired: 5 in]
        n295 = call <vilib>:"Clear Errors.vi"("error in (no error)"=w646) -> ("error out"=w637:errorcluster)  [unwired: 5 in, 1 out]
      }
      frame "Erase plot" {
        n296 = Unbundle By Name(w653) -> ("Active plot"=w652:u32)
        n297 = control-ref of="XY Graph"() -> (w648:refnum<vi>)
        n298 = case shown="3" w652 {
          tunnel: [w662 w670 w678] -> w654
          tunnel: w653 -> [w660 w668 w676]
          tunnel: w650 -> [w658 w664 w673]
          tunnel: [w657 w663 w672] -> w649
          tunnel: w648 -> [w656 w665 w671]
          frame 1, Default {
            n299 = call "measure att. peaks.vi"("First anott. index"=15, "error in"=w658, "crossovers"=dbl[] [], "XYGraph in"=w656) -> ("error out"=w657:errorcluster)  [unwired: 6 in, 1 out]
            n300 = Bundle By Name(cluster=w660, "plot 1 data"=dbl[][] []) -> (w662:T5)
          }
          frame 2 {
            n301 = call "measure att. peaks.vi"("First anott. index"=17, "error in"=w664, "crossovers"=dbl[] [], "XYGraph in"=w665) -> ("error out"=w663:errorcluster)  [unwired: 6 in, 1 out]
            n302 = Bundle By Name(cluster=w668, "plot 2 data"=dbl[][] [] ("plot 1 data")) -> (w670:T5)
          }
          frame 3 {
            n303 = call "measure att. peaks.vi"("First anott. index"=19, "error in"=w673, "crossovers"=dbl[] [], "XYGraph in"=w671) -> ("error out"=w672:errorcluster)  [unwired: 6 in, 1 out]
            n304 = Bundle By Name(cluster=w676, "plot 3 data"=dbl[][] [] ("plot 1 data")) -> (w678:T5)
          }
        }
      }
      frame "Erase all plots" {
        w679 = dbl[] []
        w684 = dbl[][] [] ("plot 1 data")
        n305 = control-ref of="XY Graph"() -> (w680:refnum<vi>)
        n306 = call "measure att. peaks.vi"("First anott. index"=15, "error in"=w688, "crossovers"=w679, "XYGraph in"=w680) -> ("error out"=w683:errorcluster)  [unwired: 6 in, 1 out]
        n307 = call "measure att. peaks.vi"("First anott. index"=17, "error in"=w683, "crossovers"=w679, "XYGraph in"=w680) -> ("error out"=w682:errorcluster)  [unwired: 6 in, 1 out]
        n308 = Bundle By Name(cluster=w690, "plot 1 data"=w684, "plot 2 data"=w684, "plot 3 data"=w684) -> (w691:T5)
        n309 = call "measure att. peaks.vi"("First anott. index"=19, "error in"=w682, "crossovers"=w679, "XYGraph in"=w680) -> ("error out"=w681:errorcluster)  [unwired: 6 in, 1 out]
      }
      frame "Save results" {
        # "Not activated"
        n310 = Write to Binary File(data=w693, error in=w695) -> (error out=w694:errorcluster)  [unwired: 4 in, 2 out]
      }
      frame "Load results" {
        w703 = T5 {"DAQmx Task Name"="", "plot 0 data (ref.)"=[], "plot 1 data"=[], "plot 2 data"=[], "plot 3 data"=[], "Anott. plots"={"plot 4 (anott.)"={"x"=[], "y"=[]}, "plot 5 (anott.)"={"x"=[], "y"=[]}, "plot 6 (anott.)"={"x"=[], "y"=[]}}, "Active plot"=0, "Recording?"=FALSE, "Cursors per plot"=0}  # App Data
        # "Not activated"
        n311 = Read from Binary File(5:w703, 8:w705) -> (0:w704:errorcluster, 2:w700:T5)  [unwired: 4 in, 2 out]
        n312 = Unbundle By Name(w700) -> ("plot 1 data"=w699:dbl[][], "plot 2 data"=w698:dbl[][], "plot 3 data"=w697:dbl[][])
        n313 = Bundle By Name(cluster=w702, "plot 1 data"=w699, "plot 2 data"=w698, "plot 3 data"=w697) -> (w701:T5)
      }
      frame "Error handler" {
        n314 = call <vilib>:"Simple Error Handler.vi"("error in (no error)"=w713) -> ("error out"=w712:errorcluster)  [unwired: 4 in, 4 out]
        n315 = call <vilib>:"Clear Errors.vi"("error in (no error)"=w712) -> ("error out"=w710:errorcluster)  [unwired: 5 in, 1 out]
        n316 = Insert Into Array(array=w709, index=0, new element=Main_Enum."Exit" ("new element/subarray")) -> (w708:T4[])
      }
      frame "Exit" {
        n317 = Unbundle By Name(w721) -> ("DAQmx Task Name"=w722:refnum<k21>)
        n318 = call <vilib>:"DAQmx Clear Task.vi"("task in"=w722, "error in"=w723) -> ("error out"=w718:errorcluster)  [unwired: 13 in]
        n319 = property class="App"(error in=w718) -> (error out=w717:errorcluster, "App.Kind"=w715:T11)  [unwired: 1 in, 1 out]
        n320 = Equal?(x=T11."Run Time System" ("y"), y=w715) -> (x = y?=w719:bool)
        n321 = case shown="True" w719 {
          frame False {
          }
          frame True {
            n322 = Quit LabVIEW() -> ()  [unwired: 1 in]
          }
        }
      }
      frame "Plot 1 cursors visibility" {
        w735 = i32[] [0, 1, 2, 3, 4, 5, 6, 7, 8, 9, 10, 11, 12]  # all anottations
        w743 = 0  # Starting cursor
        # "Cursors 0-3"
        n323 = local read "plot 1 cursors visible?"() -> (w729:bool)
        n324 = local read "Plot 1 color"() -> (w742:u32)
        n325 = control-ref of="XY Graph"() -> (w736:refnum<vi>)
        n326 = call "cursors settings.vi"("Cursor color"=w742, "Starting cursor"=w743, "error in (no error)"=w727, "Show cursors"=w729, "App Data"=w724, "XYGraph in"=w736) -> ("error out"=w738:errorcluster)  [unwired: 5 in]
        n327 = call "Curs. and anott. vis. (FGV).vi"("error in (no error)"=w738, "Enum"=T6."read") -> ("error out"=w741:errorcluster, "cursors visibility out"=w740:T10)  [unwired: 7 in, 1 out]
        n328 = Bundle By Name(cluster=w740, "plot 1 cursors visible?"=w729) -> (w739:T10)
        n329 = control-ref of="XY Graph"() -> (w733:refnum<vi>)
        n330 = call "Curs. and anott. vis. (FGV).vi"("error in (no error)"=w741, "Enum"=T6."write", "cursors visibility in"=w739) -> ("error out"=w737:errorcluster)  [unwired: 6 in, 2 out]
        n331 = call "Calculate cursors' distances.vi"("XY Graph"=w733) -> ("All cursors' dist."=w732:T16)  [unwired: 9 in, 1 out]
        n332 = local read "minimum y [dB]"() -> (w734:dbl)
        n333 = call "Update distance annotations.vi"("Y axis max"=w725, "Y axis min"=w734, "error in (no error)"=w737, "Anott. for update array in"=w735, "All cursors' dist."=w732, "XY Graph"=w736) -> ("error out"=w728:errorcluster)  [unwired: 5 in]
      }
      frame "Plot 2 cursors visibility" {
        w756 = i32[] [0, 1, 2, 3, 4, 5, 6, 7, 8, 9, 10, 11, 12]  # all anottations
        w763 = 4  # Starting cursor
        # "Cursors 4-7"
        n334 = local read "plot 2 cursors visible?"() -> (w751:bool)
        n335 = control-ref of="XY Graph"() -> (w755:refnum<vi>)
        n336 = local read "Plot 2 color"() -> (w762:u32)
        n337 = call "cursors settings.vi"("Cursor color"=w762, "Starting cursor"=w763, "error in (no error)"=w748, "Show cursors"=w751, "App Data"=w745, "XYGraph in"=w755) -> ("error out"=w758:errorcluster)  [unwired: 5 in]
        n338 = call "Curs. and anott. vis. (FGV).vi"("error in (no error)"=w758, "Enum"=T6."read") -> ("error out"=w761:errorcluster, "cursors visibility out"=w760:T10)  [unwired: 7 in, 1 out]
        n339 = Bundle By Name(cluster=w760, "plot 2 cursors visible?"=w751) -> (w759:T10)
        n340 = control-ref of="XY Graph"() -> (w754:refnum<vi>)
        n341 = call "Curs. and anott. vis. (FGV).vi"("error in (no error)"=w761, "Enum"=T6."write", "cursors visibility in"=w759) -> ("error out"=w757:errorcluster)  [unwired: 6 in, 2 out]
        n342 = call "Calculate cursors' distances.vi"("XY Graph"=w754) -> ("All cursors' dist."=w753:T16)  [unwired: 9 in, 1 out]
        n343 = local read "minimum y [dB]"() -> (w752:dbl)
        n344 = call "Update distance annotations.vi"("Y axis max"=w744, "Y axis min"=w752, "error in (no error)"=w757, "Anott. for update array in"=w756, "All cursors' dist."=w753, "XY Graph"=w755) -> ("error out"=w746:errorcluster)  [unwired: 5 in]
      }
      frame "Plot 3 cursors visibility" {
        w776 = i32[] [0, 1, 2, 3, 4, 5, 6, 7, 8, 9, 10, 11, 12]  # all anottations
        w783 = 8  # Starting cursor
        # "Cursors 8-11"
        n345 = local read "plot 3 cursors visible?"() -> (w769:bool)
        n346 = control-ref of="XY Graph"() -> (w775:refnum<vi>)
        n347 = local read "Plot 3 color"() -> (w782:u32)
        n348 = call "cursors settings.vi"("Cursor color"=w782, "Starting cursor"=w783, "error in (no error)"=w767, "Show cursors"=w769, "App Data"=w765, "XYGraph in"=w775) -> ("error out"=w781:errorcluster)  [unwired: 5 in]
        n349 = call "Curs. and anott. vis. (FGV).vi"("error in (no error)"=w781, "Enum"=T6."read") -> ("error out"=w780:errorcluster, "cursors visibility out"=w779:T10)  [unwired: 7 in, 1 out]
        n350 = Bundle By Name(cluster=w779, "plot 3 cursors visible?"=w769) -> (w778:T10)
        n351 = control-ref of="XY Graph"() -> (w774:refnum<vi>)
        n352 = call "Calculate cursors' distances.vi"("XY Graph"=w774) -> ("All cursors' dist."=w773:T16)  [unwired: 9 in, 1 out]
        n353 = call "Curs. and anott. vis. (FGV).vi"("error in (no error)"=w780, "Enum"=T6."write", "cursors visibility in"=w778) -> ("error out"=w777:errorcluster)  [unwired: 6 in, 2 out]
        n354 = local read "minimum y [dB]"() -> (w772:dbl)
        n355 = call "Update distance annotations.vi"("Y axis max"=w764, "Y axis min"=w772, "error in (no error)"=w777, "Anott. for update array in"=w776, "All cursors' dist."=w773, "XY Graph"=w775) -> ("error out"=w766:errorcluster)  [unwired: 5 in]
      }
      frame "Peak attenuation meas." {
        # "Not used"
      }
      frame "Check results (spec.)" {
        n356 = control-ref of="XY Graph"() -> (w791:refnum<vi>)
        n357 = control-ref of="Select TWT specification"() -> (w790:refnum<vi>)
        n358 = call "Check results (all plots).vi"("error in"=w794, "App Data"=w793, "XY Graph"=w791, "ComboBox in"=w790) -> ("error out"=w792:errorcluster, "results (short)"=→"Test results (spec.)":string, "detailed results"=→"detailed results":string)  [unwired: 5 in]
      }
    }
    n359 = case shown="Error" w25 {
      tunnel: w27 -> [w35 w39]
      tunnel: [w35 w38] -> w26
      frame No Error {
      }
      frame Error {
        n360 = Insert Into Array "Insert Into Array"(array=w39, index=0, new element=Main_Enum."Error handler" ("f")) -> (w38:T4[])
      }
    }
  }
  "error out 2" <- w17
